vi "TLB Native Dynamic Events ver 0.17a.vi"() -> ()   [LabVIEW 2018]
uses:
  Labview Training Phase 2/Enum Controls/States for Action Engine.ctl
  TLB Type Definitions/State Type Definitions, for 0.26d versions and later.ctl
  TLB Type Definitions/Intruction Type Definitions.ctl
  TLB Type Definitions/Encoder cluster.ctl
  TLB Type Definitions/PING CLUSTER.ctl
  <vilib>/Studica/Studica Toolkit/NavX/NavX.lvlib
  <vilib>/Studica/Studica Toolkit/Background/DIO Channel.ctl
  Underlying VI's/NavX VI/navX type def.ctl
  <vilib>/myRIO/Instrument Drivers/Utilities/Utilities.lvlib
  <vilib>/Studica/Studica Toolkit/Background/I2C Channel.ctl
  TLB Type Definitions/Vision cluster.ctl
  <vilib>/NI_Real-Time Target Support.lvlib
  TLB Type Definitions/Stepper cluster.ctl
  Experimental VI's/Archived VI's/MOTOR CONTROL NO PID Type Def.ctl
  Underlying VI's/I2C Master VI/I2C MASTER Type Def.ctl
  Underlying VI's/I2C Master VI/I2C_MASTER_WRITE_NEW Type Def.ctl
  <vilib>/userdefined/High Color/IMAQdx.ctl
  Underlying VI's/I2C Master VI/Arduino_Interfacing.ctl
  TLB Type Definitions/Yaw Cluster.ctl
  TLB Type Definitions/Time cluster.ctl
  TLB Type Definitions/Y Stepper cluster.ctl
  Underlying VI's/Modified webcam FGV/Webcam AE.ctl
  Underlying VI's/Elasped Timer/Elapsed timer control.ctl
  Underlying VI's/Motor Control VI with PID/MOTOR CONTROL WITH PID AE DATA MODE TYPE DEF.ctl
  Underlying VI's/Motor Control VI with PID/MOTOR CONTROL WITH PID AE DIRECTION TYPE DEF.ctl
  TLB Type Definitions/IR Sensor Type Def.ctl
  <vilib>/myRIO/Common/Instrument Driver Framework/myRIO v1.0/AI/typedefs/AI Channels Enum.ctl
  <vilib>/myRIO/Common/Instrument Driver Framework/myRIO v1.0/AI/typedefs/AI Channels List.ctl
  <vilib>/Utility/RT CPU Load.ctl
panel:
  out "Left IR Sensor":dbl
  out "Obstacle detected":bool
  out "Speed & distance":T1
  out "Object Center Coordinates":cluster{"x":sgl, "y":sgl}
  out "Object detection cluster":T2
  out "Time up flag":bool
  out "Task selection":u8
  in  "Object recognition mode":enum16{"Ball", "Soap", "Gel", "Pipe", "None"}(ring)
  out "NavX Readings":T3
  out "Arduino Data":T4
  out "CPU loads":T5[](array[typedef]) {"ISR (%)" format="%#.2f"; "Idle (%)" format="%#.2f"; "Background (%)" format="%#.2f"; "Normal (%)" format="%#.2f"; "Above Normal (%)" format="%#.2f"; "High (%)" format="%#.2g"; "Timed Structures (%)" format="%#.2g"; "Time Critical (%)" format="%#.2g"; "Total (%)" format="%#.2g"}
  out "TASK ENABLE":bool
  out "Rising Edge":bool
  in  "Green LED":bool
  out "I2C Error":errorcluster
  out "State Logic":T6=enum."Startup"
  out "elements":T7[](array[typedef])
  in  "STOP TASK":bool
  in  "OK Button":bool
  in  "STOP":bool
  out "error out":errorcluster
  out "Action Queue Items":i32
  out "State Logic Queue Items":i32
  out "Action Queues items":string[](array[string])=["Hardware reset", "Software reset", ""]
  out "Action State":string
  # "System Health Status Update"
  # "VISION"
  # "TLB FRAMEWORK STATUS"
  # "Test Programme written by Calvin Loke    Dated: 28 Aug 2019\nTest Programme revised by Dr Alex See   Dated 30 Aug 2019\n\nRevision date: 20/03/2020\nProgramme version:   TLB Native Dynamic Events ver 0.14a"
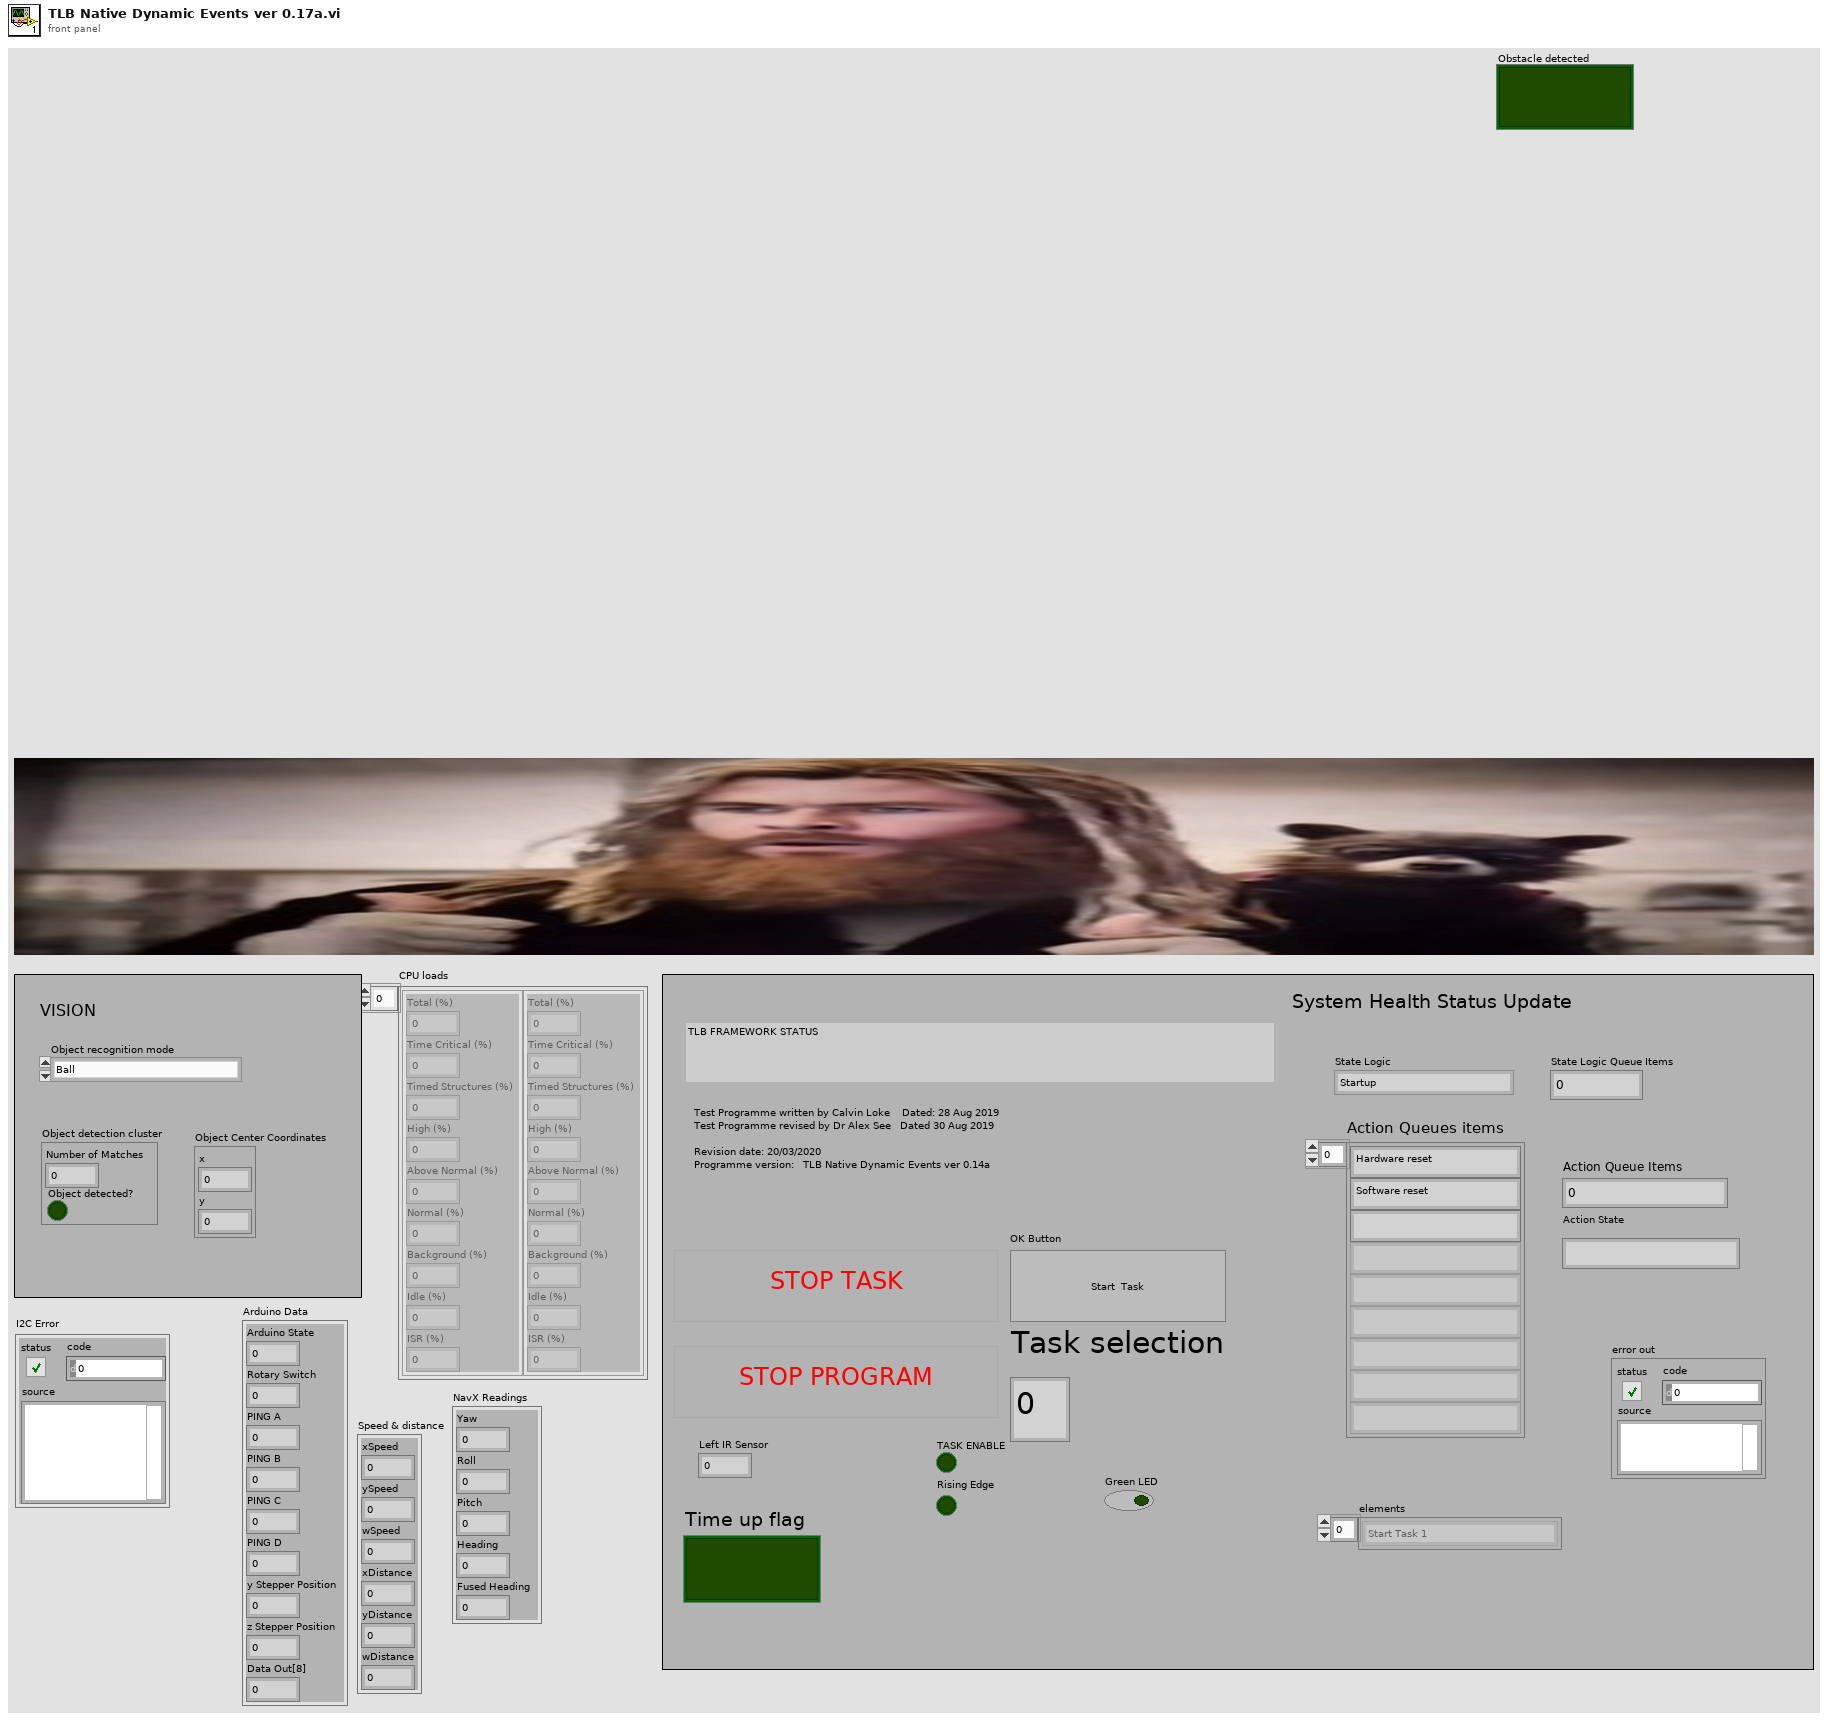
[diagram p1: front panel]
types:
  T1 = cluster{"xSpeed":dbl, "ySpeed":dbl, "wSpeed":dbl, "xDistance":dbl, "yDistance":dbl, "wDistance":dbl}
  T2 = cluster{"Number of Matches":i32, "Object detected?":bool}
  T3 = cluster{"Yaw":dbl, "Roll":dbl, "Pitch":dbl, "Heading":dbl, "Fused Heading":dbl}
  T4 = cluster{"Arduino State":u8, "Rotary Switch":u8, "PING A":u8, "PING B":u8, "PING C":u8, "PING D":u8, "y Stepper Position":u8, "z Stepper Position":u8, "Data Out[8]":u8}
  T5 = typedef "NI_Real-Time Target Support.lvlib/RT CPU Load.ctl" = cluster{"Total (%)":dbl, "Time Critical (%)":dbl, "Timed Structures (%)":dbl, "High (%)":dbl, "Above Normal (%)":dbl, "Normal (%)":dbl, "Background (%)":dbl, "Idle (%)":dbl, "ISR (%)":dbl}
  T6 = typedef "State Type Definitions.ctl" = enum16{"None", "Startup", "Move to Angle", "True Stop", "Idle", "Shutdown", "Task 1A", "Task 1B", "Task 2:Raise Arm", "Task 2:Sensor Mode", "Task 2:Reverse Mode", "Task 3", "Task 4_A", "Task 4_B", "Task 4_C", "Task 4_D", "Task 5A", "Task 5B", "Task 5C", "Task 5D", "Task 5E: POSITION ARM", "Task 5F: ARM GRAB HEIGHT", "Task 5G: CLOSE CLAW", "Task 5H: RAISE ARM", "Task 6_A", "Task 6_B", "Task 7", "Task 8A: RAISE ARM", "Task 8B: MOVE TO BOX", "Task 8C: CAM BURST", "Task 8D: PROCESS IMAGE", "Task 8E: ROBOT ADJUST", "Task 8F: CAM BURST 2", "Task 8G: PROCESS IMAGE 2", "Task 8H: ARM ADJUST", "Task 8I: ARM GRAB HEIGHT", "Task 8J: CLOSE CLAW", "Task 8K: RAISE MY SWORD", "Task 9A: Raise Arm", "Task 9B: Rotate to Angle", "Task 9C: Detect Box", "Task 9D: MOVE FORWARD", "Task 9E: MOVE LEFT", "Task 9F: SCAN IMAGE", "Task 9G: PROCESS COLOUR", "Task 9H: MOVE RIGHT", "Task 9I: SCAN IMAGE", "Task 9J: PROCESS COLOUR", "Task 9K: ROTATE 90 CW", "Task 9L: MOVE FORWARD", "Task 9M: MOVE RIGHT", "Task 9N: SCAN IMAGE", "Task 9O: PROCESS COLOUR", "Task 9P: MOVE RIGHT", "Task 9Q: SCAN IMAGE", "Task 9R: PROCESS COLOUR", "Task A1: Raise Arm", "Task A2: Rotate to Angle", "Task A3: Move Forward", "Task A4: Rotate CW 90"}
  T7 = typedef "Intruction Type Definitions.ctl" = enum16{"None", "Start Task 1", "Start Task 2", "Start Task 3", "Start Task 4", "Start Task 5", "Start Task 6", "Start Task 7", "Start Task 8 - BALL", "Start Task 8 - Gel", "Start Task 8 - Pipe", "Start Task 8 - Soap", "Start Task 9", "Start Task A", "Start Task B", "Exit"}
  T8 = typedef "IR Sensor Type Def.ctl" = cluster{"Left IR Sensor":dbl, "Arm IR Sensor":dbl, "Bottom IR Sensor":dbl}
  T9 = typedef "Y Stepper cluster.ctl" = cluster{"yStepper desired":u8}
  T10 = typedef "Time cluster.ctl" = cluster{"Time up flag":bool, "SET TIME TO CHECK":dbl}
  T11 = typedef "Yaw Cluster.ctl" = cluster{"Yaw":dbl, "Compass":dbl}
  T12 = typedef "Stepper cluster.ctl" = cluster{"y Stepper Position":u8, "z Stepper Position":u8}
  T13 = typedef "DIO Channel.ctl" = enum16{"Not Connected", "A/DIO1", "A/DIO2", "A/DIO3", "A/DIO4", "A/DIO5", "A/DIO6", "A/DIO7", "A/DIO13", "B/DIO1", "B/DIO2", "B/DIO3", "B/DIO4", "B/DIO5", "B/DIO6", "B/DIO7", "B/DIO13", "C/DIO0", "C/DIO1", "C/DIO2", "C/DIO3", "C/DIO4", "C/DIO5", "C/DIO6", "C/DIO7"}
  T14 = typedef "Vision cluster.ctl" = cluster{"Recognized Object":bool, "Object X coordinate":dbl, "Object Y coordinate":dbl}
  T15 = typedef "PING CLUSTER.ctl" = cluster{"PING_A":u8, "PING_B":u8, "PING_C":u8, "PING_D":u8}
  T16 = typedef "Encoder cluster.ctl" = cluster{"xDistance":dbl, "yDistance":dbl, "wDistance":dbl}
  T17 = cluster{"DIO Channel":T13, "FPGA VI Reference Out":refnum<k20>}
  T18 = typedef "navX type def.ctl" = enum16{"Get i2C reference", "Read Values", "Zero Yaw"}
  T19 = typedef "Arduino_Interfacing.ctl" = enum16{"Initialize", "Write to Arduino", "Read From Arduino"}
  T20 = typedef "I2C Channel.ctl" = enum16{"Not Connected", "A", "B"}
  T21 = typedef "States for Action Engine.ctl" = enum16{"Initialize", "Write", "Read"}
  T22 = cluster{"I2C Ref Out":cluster{"I2C Channel":T20, "FPGA VI Reference Out":refnum<k20>}, "Connected":bool, "Slave Address (7-bit)":u8, "Registry":u8[]}
  T23 = typedef "IMAQ Image.ctl" = refnum<image>
  T24 = typedef "State Type Definitions.ctl" = enum16{"None", "Startup", "Move to Angle", "True Stop", "Idle", "Shutdown", "Task 1", "Task 2:Raise Arm", "Task 2:Sensor Mode", "Task 2:Reverse Mode", "Task 3", "Task 4_A", "Task 4_B", "Task 4_C", "Task 4_D", "Task 5_A", "Task 5 _B", "Task 5_C", "Task 5_D", "Task 5_D_Error", "Task 5D_Error_Right", "Task 5D_Error_Left", "Task 5_E", "Task 5_F", "Task 5F_Error", "Task 5G", "Task 5H", "Task 5I", "Task 6_A", "Task 6_B", "Task 7", "Task 8", "Task 9A: Raise Arm", "Task 9B: Rotate to Angle", "Task 9C: Rotation alignmnet", "Task B"}
  T25 = typedef "MOTOR CONTROL WITH PID AE DIRECTION TYPE DEF.ctl" = enum16{"y-axis movement", "x-axis movement", "rotation", "stop", "reset encoders"}
  T26 = typedef "MOTOR CONTROL WITH PID AE DATA MODE TYPE DEF.ctl" = enum16{"Init AE", "Write to AE", "Read from AE"}
  T27 = typedef "Elapsed timer control.ctl" = enum16{"Start", "Pause", "Initialize"}
  T28 = typedef "I2C_MASTER_WRITE_NEW Type Def.ctl" = enum16{"Ultrasonic sensors", "Stepper origin", "zStepper 13.3k", "zStepper 13k", "zStepper 12k", "zStepper 11k", "zStepper 10k", "zStepper 9k", "zStepper 8k", "zStepper 7k", "zStepper 6k", "zStepper 5k", "zStepper 4k", "zStepper 3k", "zStepper 2k", "zStepper 1k", "zStepper 900", "zStepper 800", "zStepper 700", "zStepper 600", "zStepper 500", "zStepper 400", "zStepper 300", "zStepper 200", "zStepper 100", "zStepper 0", "yStepper control", "Open Claw", "Close Claw", "Soft Reset"}
  T29 = typedef "Webcam AE.ctl" = enum16{"Initialize Camera", "Open Camera", "Continuous Acquisition", "Close Camera", "Retrieve Image", "Dispose Camera Image Buffer"}
  T30 = typedef "IMAQdx.ctl" = refnum<k21>
  T31 = typedef "Webcam AE.ctl" = enum16{"Initialize Camera", "Open Camera", "Continuous Acquisition", "Close Camera", "Retrieve Image", "Dispose Image Buffers"}
  T32 = typedef "MOTOR CONTROL NO PID Type Def.ctl" = enum16{"Init", "Front Back", "Left Right", "Rotate", "Stop", "Latch"}
  T33 = typedef "AI Channels List.ctl" = T34[]
  T34 = typedef "AI Channels Enum.ctl" = enum16{"Not Connected", "AudioIn/Left", "AudioIn/Right", "C/AI0", "C/AI1", "A/AI0", "A/AI1", "A/AI2", "A/AI3", "A/AI4", "A/AI5", "A/AI6", "A/AI7", "B/AI0", "B/AI1", "B/AI2", "B/AI3", "B/AI4", "B/AI5", "B/AI6", "B/AI7", "AI/AI0", "AI/AI1", "AI/AI2", "AI/AI3", "A/AI0 (DIFF)", "A/AI1 (DIFF)", "A/AI2 (DIFF)", "A/AI3 (DIFF)", "B/AI0 (DIFF)", "B/AI1 (DIFF)", "B/AI2 (DIFF)", "B/AI3 (DIFF)"}
  T35 = typedef "I2C MASTER Type Def.ctl" = enum16{"Last State", "Mode 0", "Mode 1", "Mode 2", "Mode 3", "Mode 4", "Mode 5", "Mode 6", "Mode 7", "Mode 8", "Mode 9", "Mode 10"}
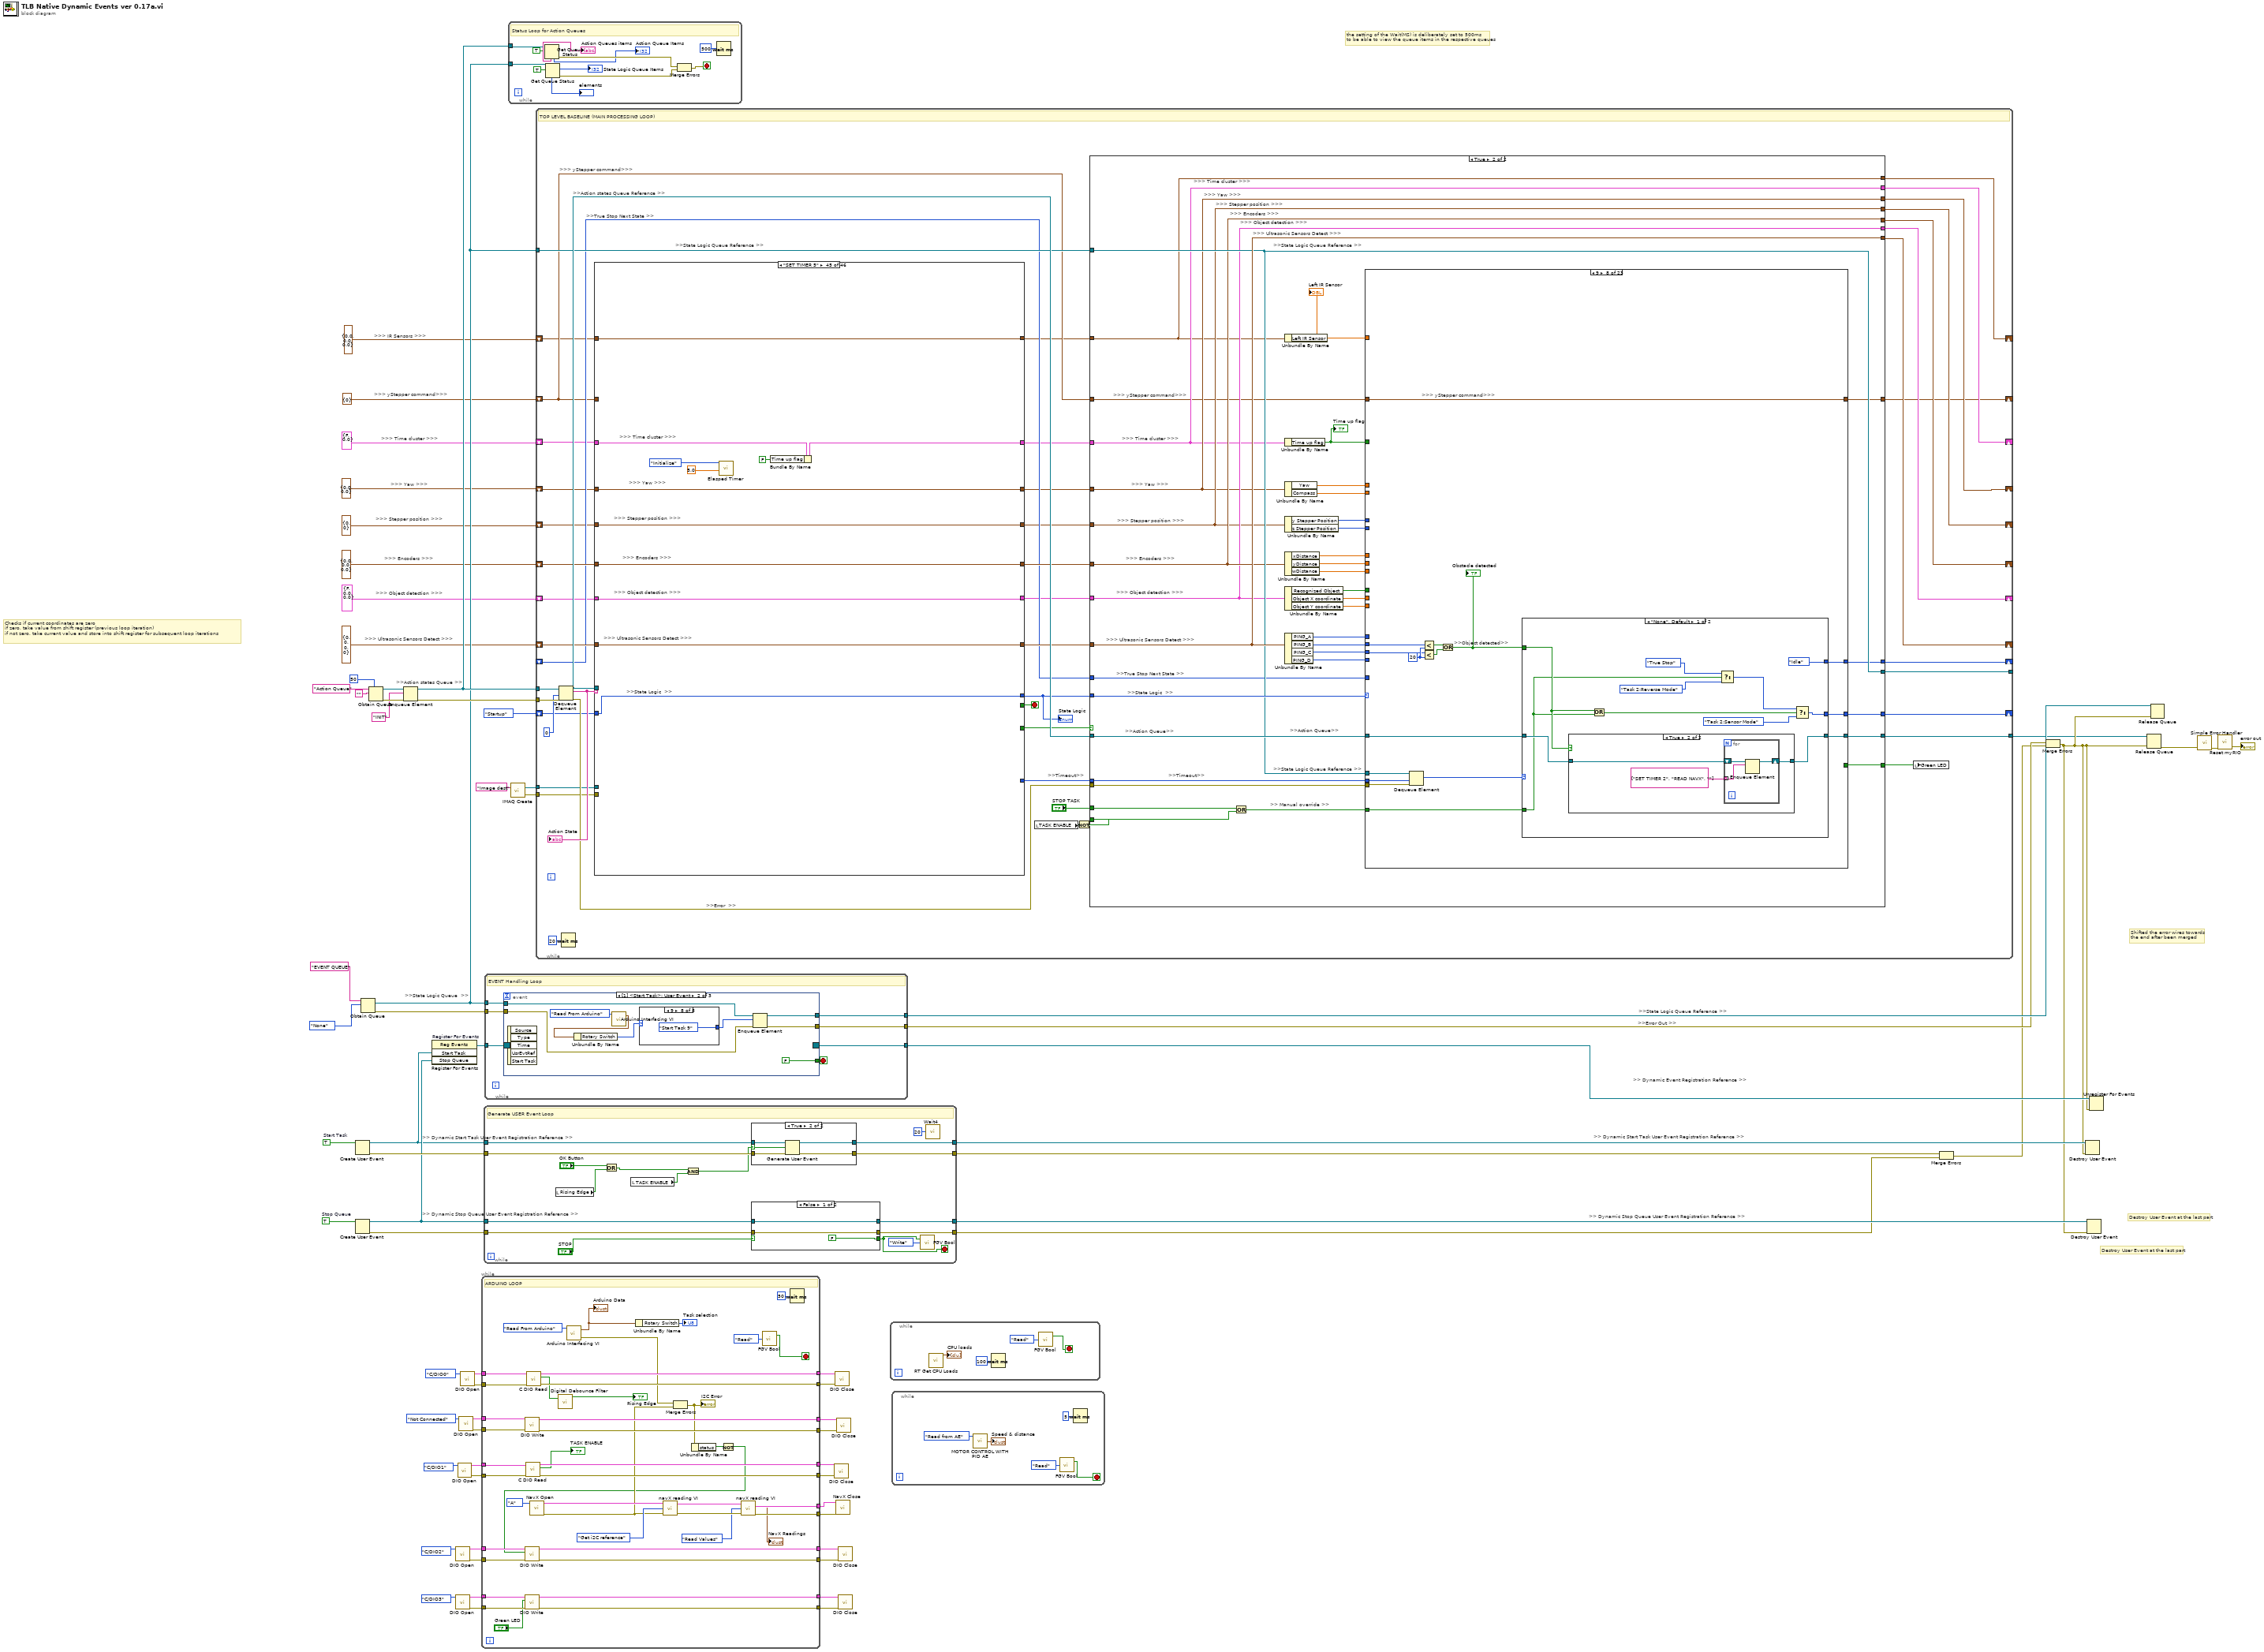
[diagram p0: block diagram]
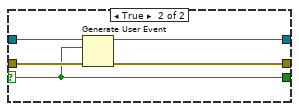
[diagram p2: hidden frame]
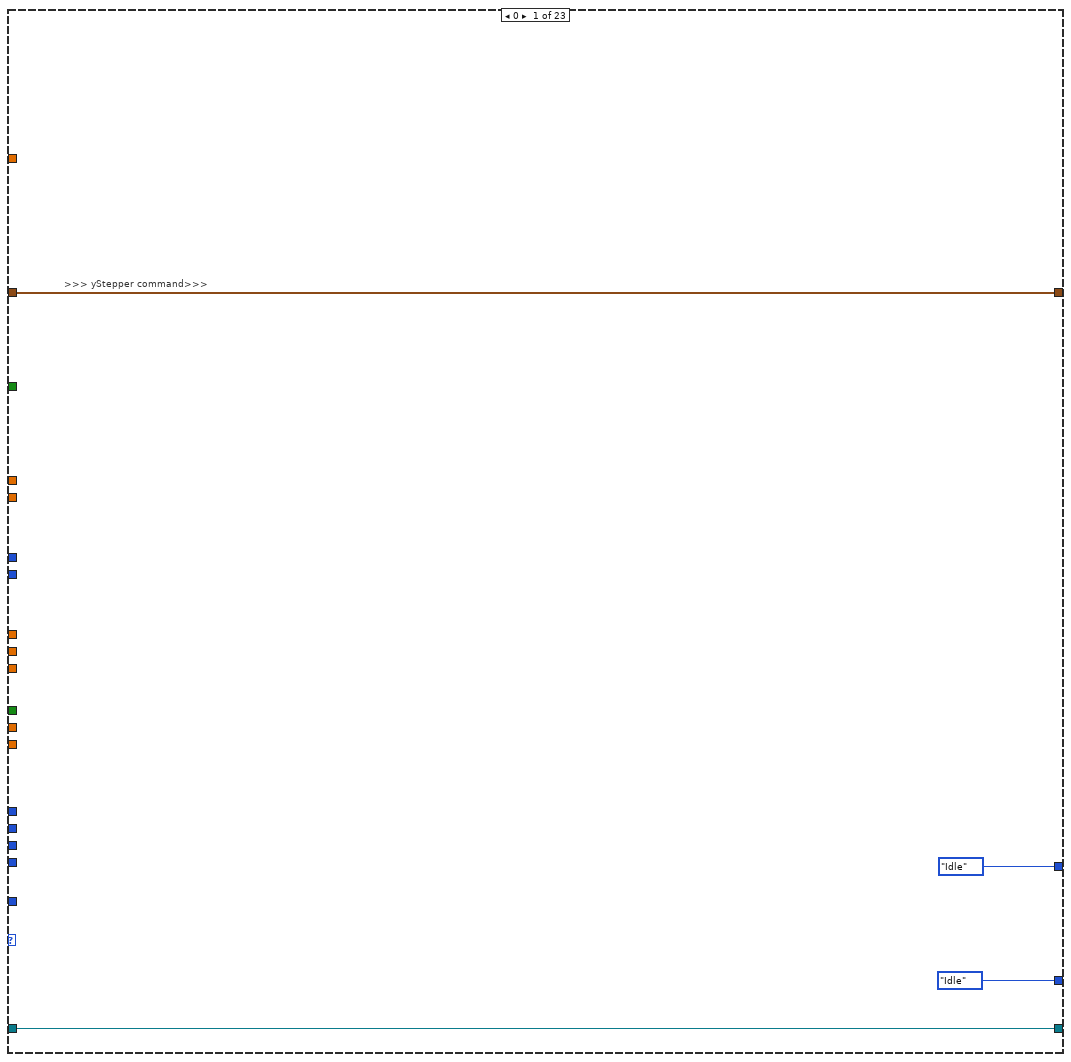
[diagram p5: hidden frame]
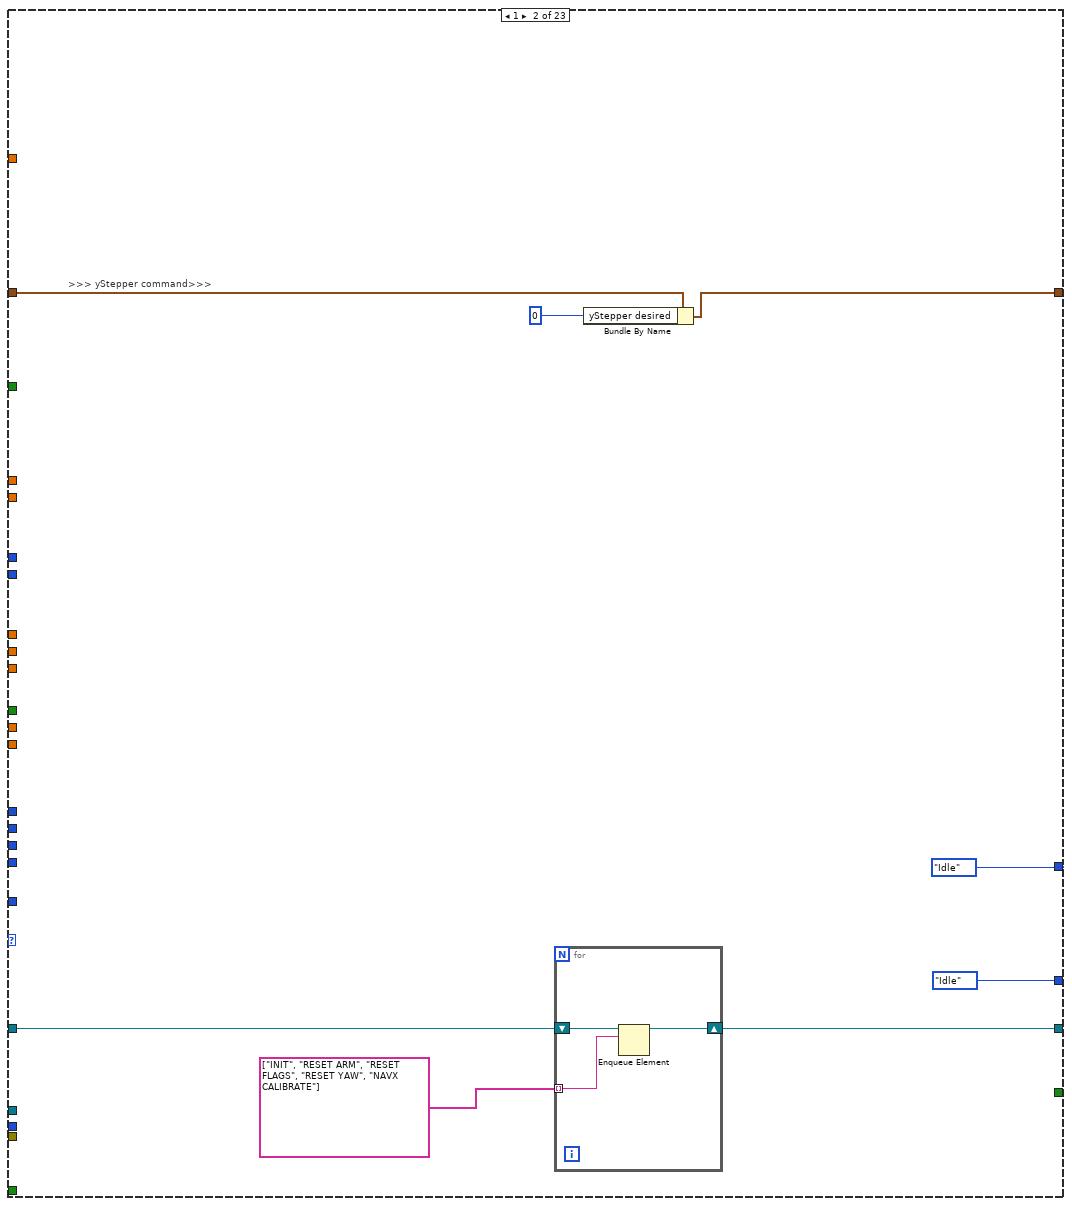
[diagram p6: hidden frame]
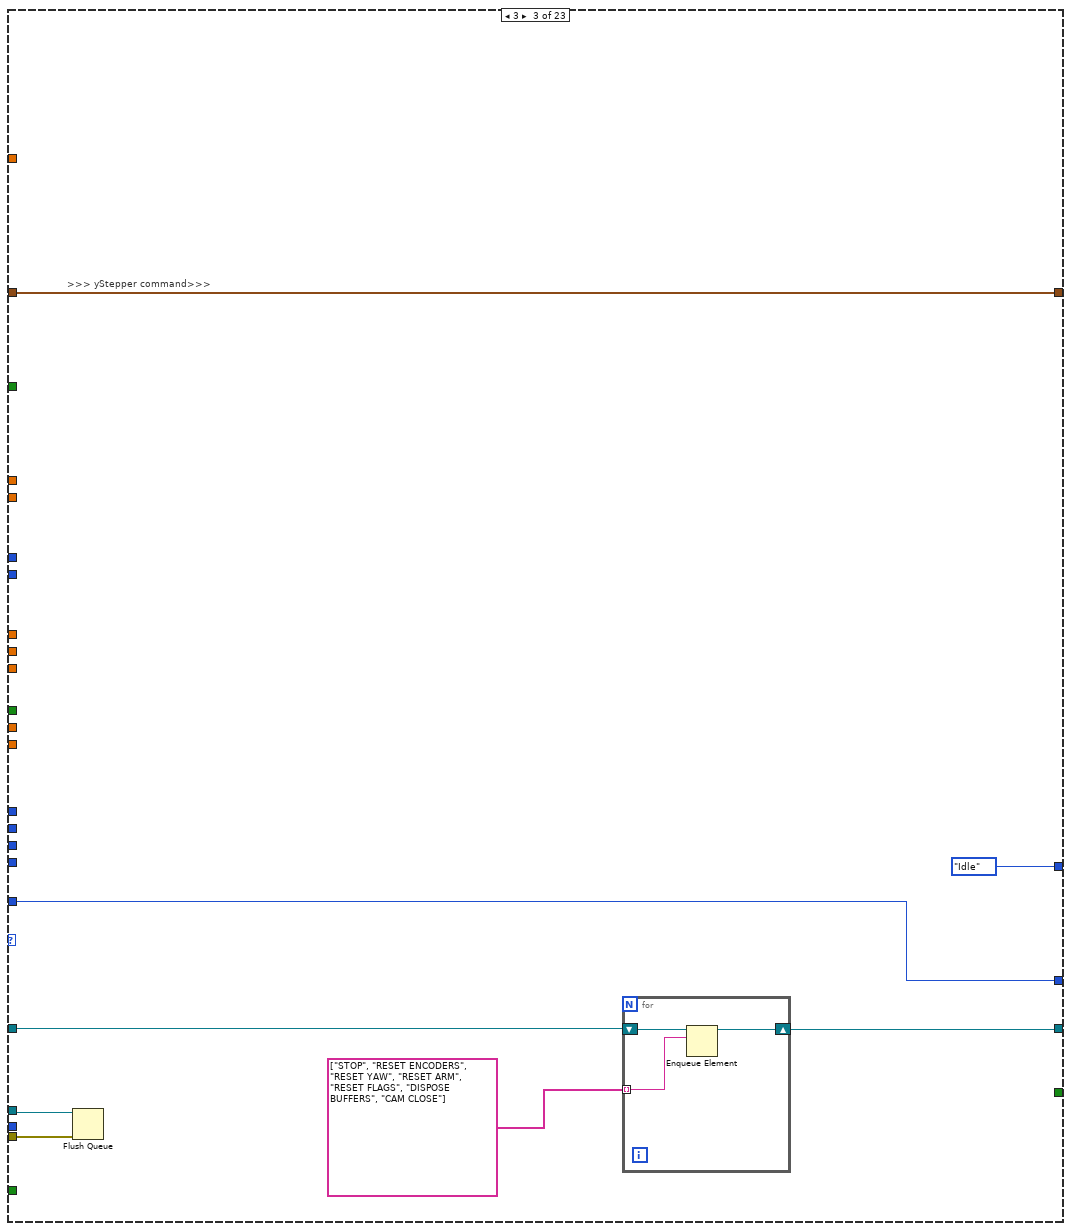
[diagram p7: hidden frame]
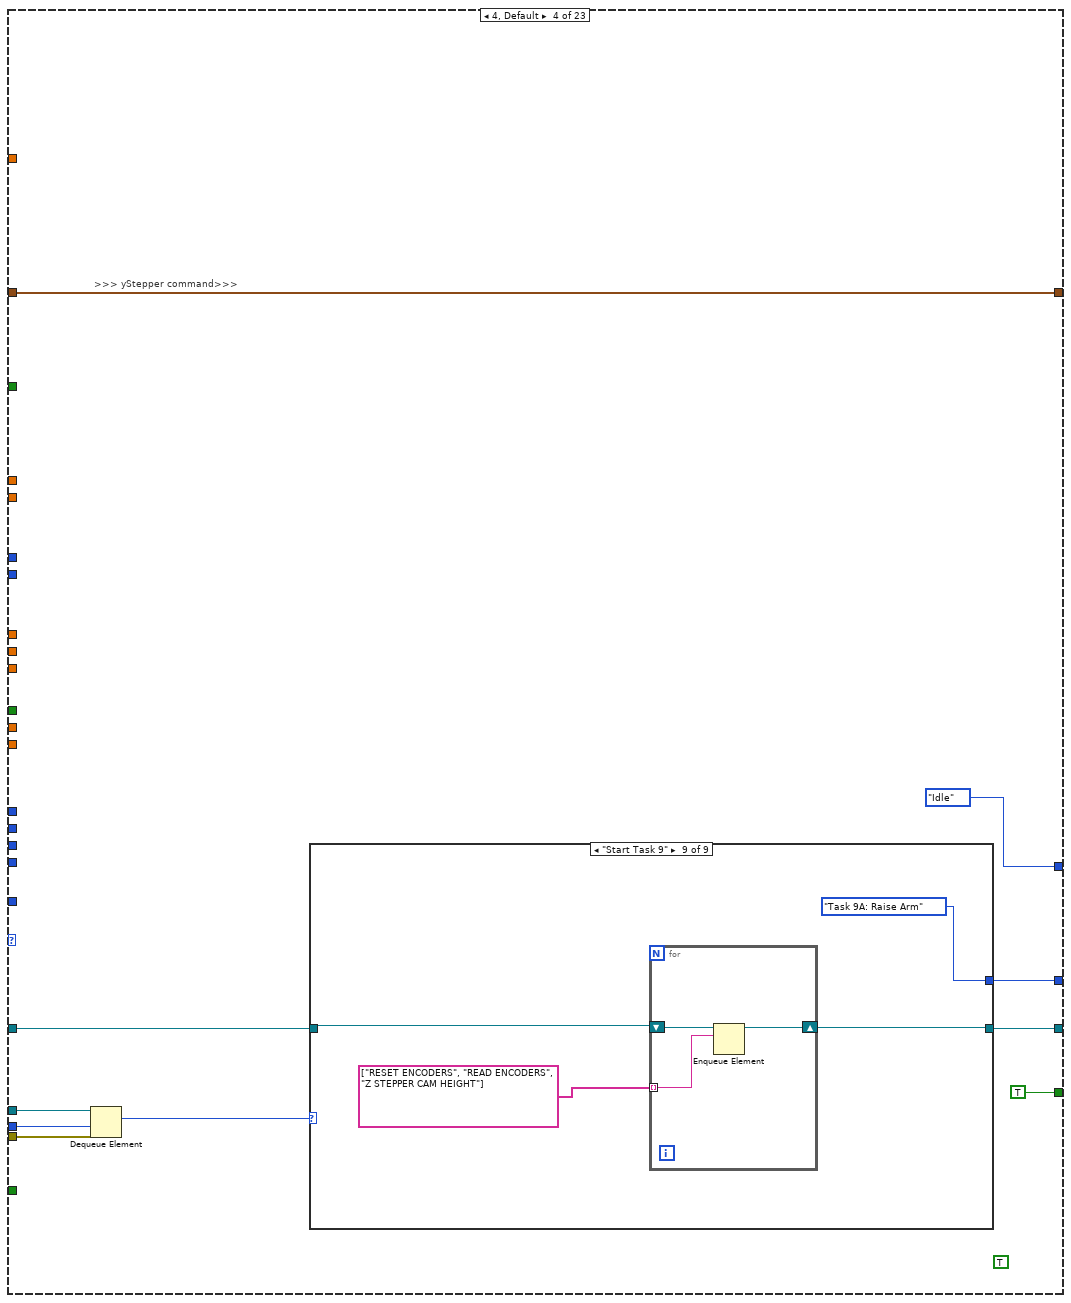
[diagram p8: hidden frame]
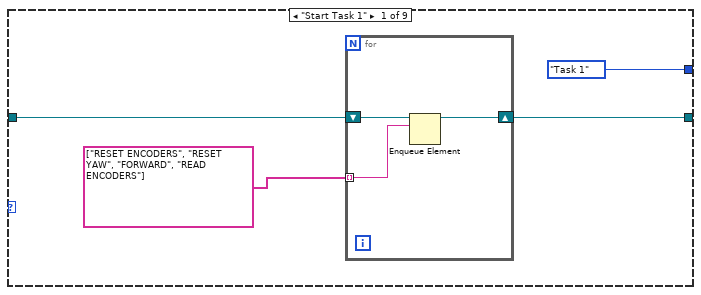
[diagram p9: hidden frame]
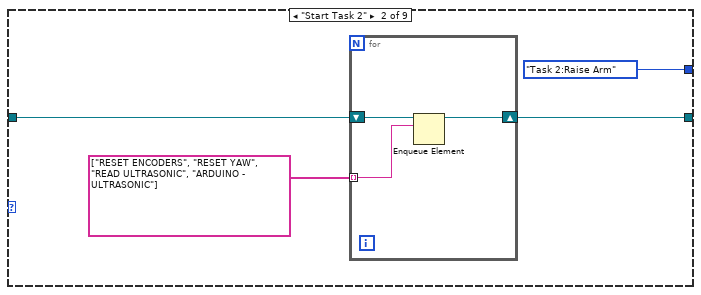
[diagram p10: hidden frame]
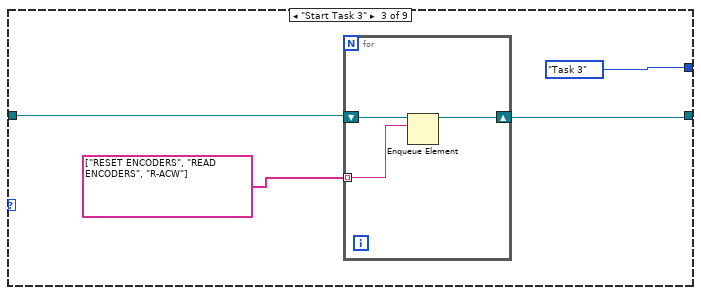
[diagram p11: hidden frame]
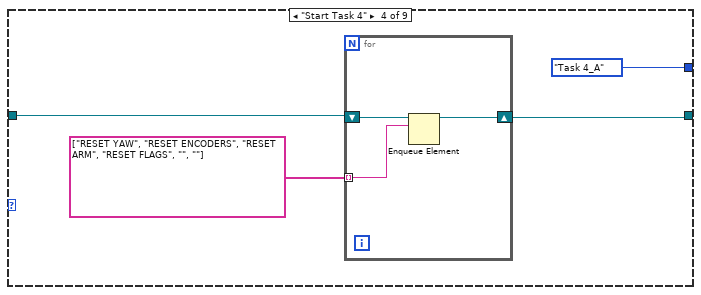
[diagram p12: hidden frame]
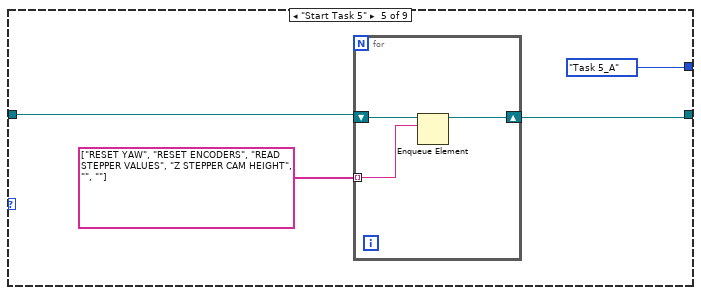
[diagram p13: hidden frame]
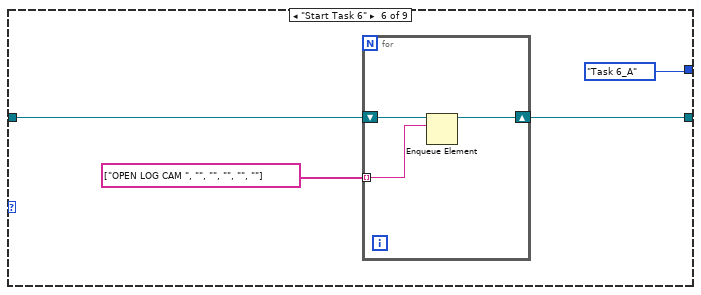
[diagram p14: hidden frame]
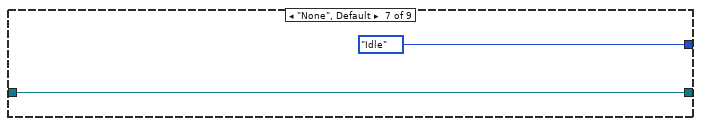
[diagram p15: hidden frame]
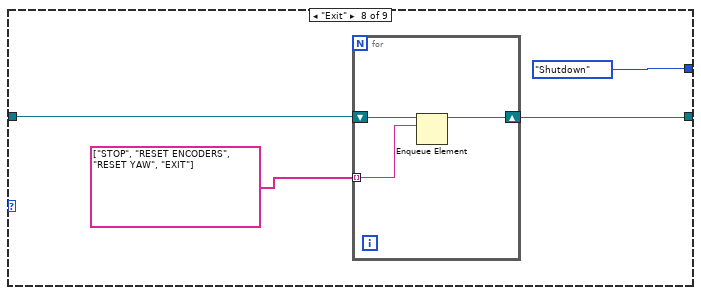
[diagram p16: hidden frame]
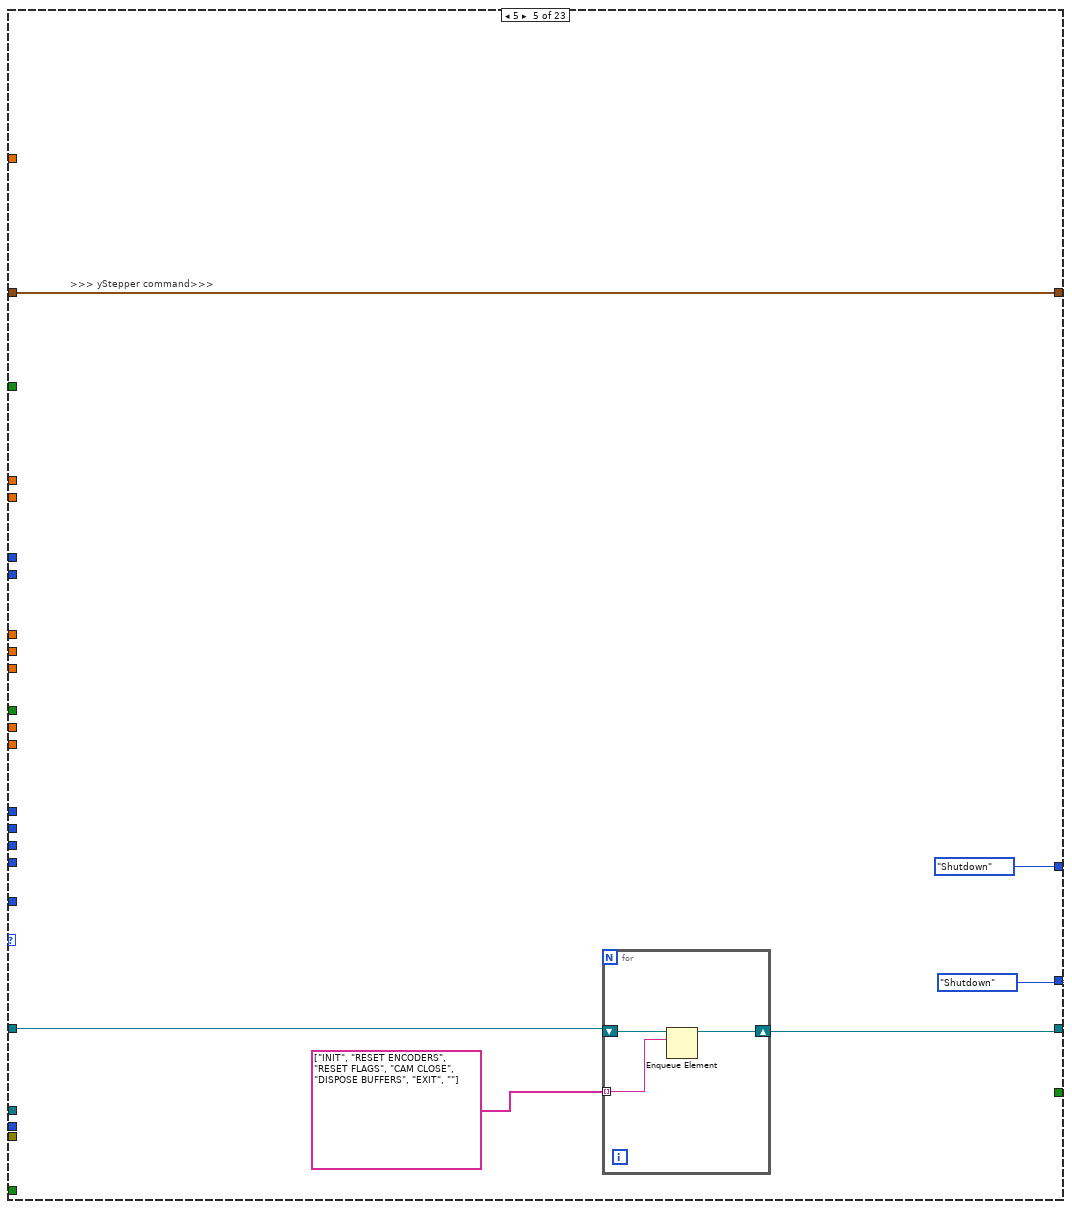
[diagram p17: hidden frame]
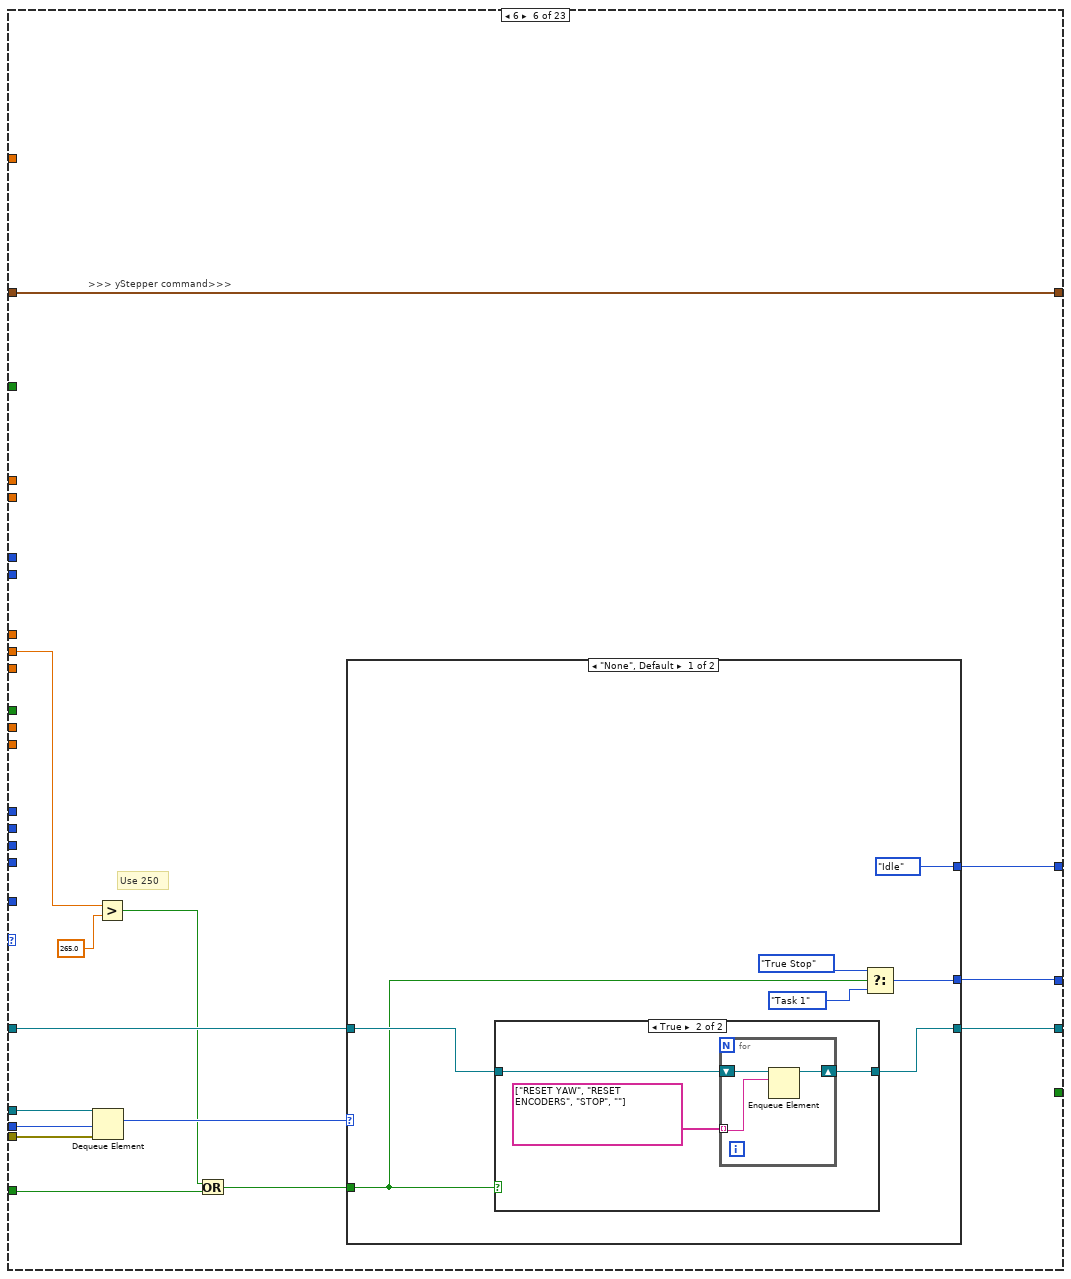
[diagram p18: hidden frame]
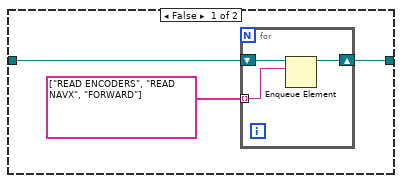
[diagram p19: hidden frame]
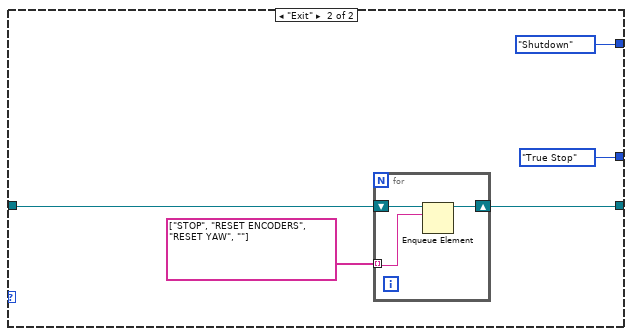
[diagram p20: hidden frame]
diagram:
  w71 = TRUE  # Stop Queue
  w70 = TRUE  # Start Task
  # ">>> IR Sensors >>>"
  # "Checks if current coordinates are zero\nif zero, take value from shift register (previous loop iteration)\nif not zero, take current value and store into shift register for subsequent loop iterations"
  # ">>> yStepper command>>>"
  # ">>> Time cluster >>>"
  # ">>> Yaw >>>"
  # ">>> Stepper position >>>"
  # ">>> Encoders >>>"
  # ">>> Object detection >>>"
  # ">>> Ultrasonic Sensors Detect >>>"
  # "the setting of the Wait(MS) is deliberately set to 500ms\nto be able to view the queue items in the respective queues"
  # ">>Error Out >>"
  # ">> Dynamic Stop Queue User Event Registration Reference >>"
  # ">> Dynamic Start Task User Event Registration Reference >>"
  # ">> Dynamic Stop Queue User Event Registration Reference >>"
  # ">> Dynamic Start Task User Event Registration Reference >>"
  # ">> Dynamic Event Registration Reference >>"
  # ">>Action states Queue >>"
  # ">>State Logic Queue  >>"
  # ">>State Logic Queue Reference >>"
  # "Destroy User Event at the last part"
  # "Destroy User Event at the last part"
  # "Shifted the error wires towards\nthe end after been merged"
  n1 = Create User Event(user event datatype=w70) -> (user event=w62:refnum<user-event>, error out=w67:errorcluster)  [unwired: 1 in]
  n2 = Create User Event(user event datatype=w71) -> (user event=w63:refnum<user-event>, error out=w66:errorcluster)  [unwired: 1 in]
  n3 = Obtain Queue(name (unnamed)="EVENT QUEUE", element data type=Intruction_Type_Definitions."None" ("Enum")) -> (queue out=w48:refnum<queue>, error out=w54:errorcluster)  [unwired: 3 in, 1 out]
  n4 = Obtain Queue(max queue size (-1, unlimited)=50, name (unnamed)="Action Queue", element data type="") -> (queue out=w57:refnum<queue>, error out=w53:errorcluster)  [unwired: 2 in, 1 out]
  n5 = Enqueue Element(queue=w57, element="INIT", error in (no error)=w53) -> (queue out=w49:refnum<queue>, error out=w52:errorcluster)  [unwired: 1 in, 1 out]
  n6 = register-events "Register For Events"(w62, w63) -> (reference out=w61:refnum<event-registration>)  [unwired: 2 in, 1 out]
  n7 = call <vilib>:"DIO Open.vi"("DIO Channel"=DIO_Channel."C/DIO2") -> ("error out"=w15:errorcluster, "DIO Info Out"=w16:T17)  [unwired: 9 in]
  n8 = call <vilib>:"DIO Open.vi"("DIO Channel"=DIO_Channel."C/DIO3") -> ("error out"=w10:errorcluster, "DIO Info Out"=w11:T17)  [unwired: 9 in]
  n9 = call <vilib>:"DIO Open.vi"("DIO Channel"=DIO_Channel."C/DIO1") -> ("error out"=w26:errorcluster, "DIO Info Out"=w27:T17)  [unwired: 9 in]
  n10 = call <vilib>:"DIO Open.vi"("DIO Channel"=DIO_Channel."Not Connected") -> ("error out"=w31:errorcluster, "DIO Info Out"=w33:T17)  [unwired: 9 in]
  n11 = call <vilib>:"DIO Open.vi"("DIO Channel"=DIO_Channel."C/DIO0") -> ("error out"=w36:errorcluster, "DIO Info Out"=w39:T17)  [unwired: 9 in]
  n12 = while {
    tunnel: w39 -> [w112]
    tunnel: [w111] -> w37
    tunnel: w36 -> [w110]
    tunnel: [w109] -> w35
    tunnel: w33 -> [w106]
    tunnel: [w105] -> w32
    tunnel: w31 -> [w104]
    tunnel: [w103] -> w30
    tunnel: [w102] -> w28
    tunnel: w27 -> [w101]
    tunnel: w26 -> [w100]
    tunnel: [w99] -> w25
    tunnel: w16 -> [w93]
    tunnel: w15 -> [w92]
    tunnel: [w91] -> w14
    tunnel: [w90] -> w13
    tunnel: w11 -> [w89]
    tunnel: w10 -> [w88]
    tunnel: [w87] -> w9
    tunnel: [w86] -> w8
    tunnel: [w80] -> w5
    tunnel: [w79] -> w6
    stop <- w114 stop-if-true
    # "ARDUINO LOOP"
    n13 = call <vilib>:"DIO Write.vi"("error in (no error)"=w88, "Input"="Green LED", "DIO Info In"=w89) -> ("error out"=w86:errorcluster, "DIO Info Out"=w87:T17)  [unwired: 7 in]
    n14 = call <vilib>:"DIO Write.vi"("error in (no error)"=w104, "DIO Info In"=w106) -> ("error out"=w103:errorcluster, "DIO Info Out"=w105:T17)  [unwired: 8 in]
    n15 = call <vilib>:"C DIO Read.vi"("error in (no error)"=w100, "DIO Info In in"=w101) -> ("error out"=w99:errorcluster, "IN"=→"TASK ENABLE":bool, "DIO Info In out"=w102:T17)  [unwired: 7 in]
    n16 = call <vilib>:"C DIO Read.vi"("error in (no error)"=w110, "DIO Info In in"=w112) -> ("error out"=w109:errorcluster, "IN"=w108:bool, "DIO Info In out"=w111:T17)  [unwired: 7 in]
    n17 = call <vilib>:"NavX Open.vi"("I2C Channel"=I2C_Channel."A") -> ("error out"=w95:errorcluster, "NavX Info"=w97:T22)  [unwired: 9 in]
    n18 = call "Digital Debounce Filter.vi"("Boolean input"=w108) -> ("Rising Edge"=→"Rising Edge":bool)  [unwired: 1 in, 2 out]
    n19 = call "Arduino Interfacing VI.vi"("AE Mode"=Arduino_Interfacing."Read From Arduino") -> ("error out"=w83:errorcluster, "Arduino Data"=w76:T4)  [unwired: 3 in]
    "Arduino Data" <- w76
    n20 = Unbundle By Name(w76) -> ("Rotary Switch"=→"Task selection":u8)
    n21 = call "navX reading VI.vi"("NavX Info In"=w97, "Mode"=navX_type_def."Get i2C reference", "error in (no error)"=w95) -> ("NavX Info Out"=w82:T22, "Error Out"=w81:errorcluster)  [unwired: 2 out]
    n22 = Merge Errors(w83, w95) -> (w74:errorcluster)
    "I2C Error" <- w74
    n23 = Unbundle By Name(w74) -> ("status"=w73:bool)
    n24 = Not(x=w73) -> (.not. x?=w72:bool)
    n25 = call <vilib>:"DIO Write.vi"("error in (no error)"=w92, "Input"=w72, "DIO Info In"=w93) -> ("error out"=w90:errorcluster, "DIO Info Out"=w91:T17)  [unwired: 7 in]
    n26 = call "navX reading VI.vi"("NavX Info In"=w82, "Mode"=navX_type_def."Read Values", "error in (no error)"=w81) -> ("NavX Info Out"=w80:T22, "NavX Readings"=→"NavX Readings":T3, "Error Out"=w79:errorcluster)  [unwired: 1 out]
    n27 = call "FGV Bool.vi"("Init/Read/Write State"=States_for_Action_Engine."Read") -> ("Output node"=w114:bool)  [unwired: 2 in, 1 out]
    n28 = Wait (ms)(milliseconds to wait=u32 50) -> ()  [unwired: 1 out]
  }
  n29 = while {
    tunnel: w62 -> [w132]
    tunnel: w63 -> [w131]
    tunnel: [w130] -> w69
    tunnel: [w129] -> w68
    tunnel: w67 -> [w128]
    tunnel: [w127] -> w65
    tunnel: w66 -> [w126]
    tunnel: [w125] -> w64
    stop <- w123 stop-if-true
    # "Generate USER Event Loop"
    n30 = local read "Rising Edge"() -> (w119:bool)
    n31 = Or(x="OK Button", y=w119) -> (x .or. y?=w118:bool)
    n32 = local read "TASK ENABLE"() -> (w117:bool)
    n33 = And(x=w118, y=w117) -> (x .and. y?=w116:bool)
    n34 = case shown="True" w116 {
      selector: w116 -> [_ w143]
      tunnel: w132 -> [w142 w147]
      tunnel: [w142 w146] -> w129
      tunnel: w128 -> [w141 w145]
      tunnel: [w141 w144] -> w127
      frame False {
      }
      frame True {
        n35 = Generate User Event(user event=w147, event data cluster=w143, error in=w145) -> (user event out=w146:refnum<user-event>, error out=w144:errorcluster)  [unwired: 1 in]
      }
    }
    n36 = case shown="False" "STOP" {
      selector: "STOP" -> [_ w136]
      tunnel: w131 -> [w135 w140]
      tunnel: [w135 w139] -> w130
      tunnel: w126 -> [w134 w138]
      tunnel: [w134 w137] -> w125
      tunnel: [FALSE w136] -> w123
      frame False {
      }
      frame True {
        n37 = Generate User Event(user event=w140, event data cluster=w136, error in=w138) -> (user event out=w139:refnum<user-event>, error out=w137:errorcluster)  [unwired: 1 in]
      }
    }
    n38 = call "FGV Bool.vi"("Init/Read/Write State"=States_for_Action_Engine."Write", "Input Node"=w123) -> ()  [unwired: 1 in, 2 out]
    n39 = call "Wait4"("Count(uSec)"=u32 20) -> ()  [unwired: 1 out]
  }
  n40 = while {
    tunnel: w61 -> [w154]
    tunnel: [w153] -> w60
    tunnel: w48 -> [w151]
    tunnel: [w150] -> w59
    tunnel: w54 -> [w149]
    tunnel: [w148] -> w51
    stop <- w152 stop-if-true
    # "EVENT Handling Loop"
    n41 = event shown="[1] <Start Task>: User Event" {
      selector: w154 -> [_ _ _]
      dyn-events: [_ _ _] -> w153
      timeout: _ -> [_ _ _]
      tunnel: [FALSE FALSE w183] -> w152
      tunnel: w151 -> [w159 w168 w181]
      tunnel: [w158 w167 w182] -> w150
      tunnel: w149 -> [w157 w166 w180]
      tunnel: [w156 w165 w179] -> w148
      event Timeout {
        n42 = event-data() -> ()  [unwired: 1 in, 3 out]
        n43 = Enqueue Element(queue=w159, element=Intruction_Type_Definitions."None" ("Enum"), error in (no error)=w157) -> (queue out=w158:refnum<queue>, error out=w156:errorcluster)  [unwired: 1 in, 1 out]
      }
      event User Event {
        n44 = event-data() -> ()  [unwired: 1 in, 5 out]
        n45 = call "Arduino Interfacing VI.vi"("AE Mode"=Arduino_Interfacing."Read From Arduino") -> ("Arduino Data"=w162:T4)  [unwired: 3 in, 1 out]
        n46 = Unbundle By Name(w162) -> ("Rotary Switch"=w161:u8)
        n47 = case shown="9" w161 {
          tunnel: [Intruction_Type_Definitions."None" ("Enum") Intruction_Type_Definitions."Start Task 1" ("Enum") Intruction_Type_Definitions."Start Task 2" ("Enum") Intruction_Type_Definitions."Start Task 3" ("Enum") Intruction_Type_Definitions."Start Task 4" ("Enum") Intruction_Type_Definitions."Start Task 5" ("Enum") Intruction_Type_Definitions."Start Task 6" ("Enum") Intruction_Type_Definitions."Start Task 9" ("Enum")] -> w164
          frame 0, Default {
          }
          frame 1 {
          }
          frame 2 {
          }
          frame 3 {
          }
          frame 4 {
          }
          frame 5 {
          }
          frame 6 {
          }
          frame 9 {
          }
        }
        n48 = Enqueue Element(queue=w168, element=w164, error in (no error)=w166) -> (queue out=w167:refnum<queue>, error out=w165:errorcluster)  [unwired: 1 in, 1 out]
      }
      event User Event {
        n49 = event-data() -> ("Stop Queue"=w183:bool)  [unwired: 1 in, 4 out]
        n50 = Enqueue Element At Opposite End(queue=w181, element=Intruction_Type_Definitions."Exit" ("Enum"), error in (no error)=w180) -> (queue out=w182:refnum<queue>, error out=w179:errorcluster)  [unwired: 1 in, 1 out]
      }
    }
  }
  n51 = while {
    tunnel: w49 -> [w193]
    tunnel: w48 -> [w190]
    stop <- w187 stop-if-true
    # "Status Loop for Action Queues"
    n52 = Get Queue Status(queue=w193, return elements? (F)=TRUE) -> (error out=w189:errorcluster, # elements in queue=→"Action Queue Items":i32, elements=→"Action Queues items":string[])  [unwired: 1 in, 5 out]
    n53 = Get Queue Status(queue=w190, return elements? (F)=TRUE) -> (# pending remove=→"State Logic Queue Items":i32, error out=w188:errorcluster, elements=→"elements":T7[])  [unwired: 1 in, 5 out]
    n54 = Merge Errors(w189, w188) -> (w187:errorcluster)
    n55 = Wait (ms)(milliseconds to wait=u32 500) -> ()  [unwired: 1 out]
  }
  n56 = call "IMAQ Create"("Image Name"="Image dest") -> ("New Image"=w20:T23, "error out"=w19:errorcluster)  [unwired: 4 in]
  n57 = while {
    tunnel: w48 -> [w230]
    tunnel: w49 -> [w242]
    tunnel: w52 -> [w240]
    tunnel: [w239] -> _
    tunnel: [w238] -> w42
    shift-right: [w231] -> _
    shift-left: T15 {"PING_A"=0, "PING_B"=0, "PING_C"=0, "PING_D"=0} -> [w233]
    shift-right: [w224] -> _
    shift-left: State_Type_Definitions."Startup" ("Enum") -> [w227]
    shift-right: [w220] -> _
    shift-left: T16 {"xDistance"=0.0, "yDistance"=0.0, "wDistance"=0.0} -> [w222]
    shift-right: [w217] -> _
    shift-left: _ -> [w216]
    tunnel: w20 -> [w215]
    tunnel: w19 -> [w214]
    shift-right: [w211] -> _
    shift-left: T14 {"Recognized Object"=FALSE, "Object X coordinate"=0.0, "Object Y coordinate"=0.0} -> [w213]
    shift-right: [w208] -> _
    shift-left: T12 {"y Stepper Position"=0, "z Stepper Position"=0} -> [w210]
    shift-right: [w205] -> _
    shift-left: T11 {"Yaw"=0.0, "Compass"=0.0} -> [w207]
    shift-right: [w202] -> _
    shift-left: T10 {"Time up flag"=FALSE, "SET TIME TO CHECK"=0.0} -> [w204]
    shift-right: [w200] -> _
    shift-left: T9 {"yStepper desired"=0} -> [w201]
    shift-right: [w196] -> _
    shift-left: T8 {"Left IR Sensor"=0.0, "Arm IR Sensor"=0.0, "Bottom IR Sensor"=0.0} -> [w198]
    stop <- w229 stop-if-true
    # ">>> yStepper command>>>"
    # ">>True Stop Next State >>"
    # ">>Error  >>"
    # ">>Timeout>>"
    # ">>Action states Queue Reference >>"
    # ">>State Logic Queue Reference >>"
    # "TOP LEVEL BASELINE (MAIN PROCESSING LOOP)"
    n58 = Dequeue Element(queue=w242, timeout in ms (-1)=0, error in (no error)=w240) -> (queue out=w234:refnum<queue>, element=w241:string, error out=w235:errorcluster)  [unwired: 1 out]
    "Action State" <- w241
    n59 = Wait (ms)(milliseconds to wait=u32 20) -> ()  [unwired: 1 out]
    n60 = case shown="\"SET TIMER 5\"" w241 {
      tunnel: [_ _ _ _ _ _ _ _ _ _ _ _ _ _ _ _ _ _ 0 w1421 _ _ _ _ _ _ _ _ _ _ _ _ _ _ _ _ _ _ _ _ _ _ _ _ _ _] -> w237
      tunnel: w234 -> [_ _ _ _ _ _ _ _ _ _ _ _ _ _ _ _ _ _ _ _ _ _ _ _ _ _ _ _ _ _ _ _ _ _ _ _ _ _ _ _ _ _ _ _ _ _]
      tunnel: w233 -> [w1192 w1201 w1213 w1224 w1241 w1252 w1263 w1275 w1287 w1298 w1305 w1320 w1334 w1346 w1354 w1366 w1391 w1401 w1412 w1422 w1431 w1441 w1471 w1482 w1490 w1499 w1512 w1525 w1535 w1544 w1561 w1570 w1581 w1591 w1601 w1611 w1618 w1630 w1646 w1652 w1664 w1676 w1688 w1700 w1712 w1723]
      tunnel: [w1192 w1201 w1213 w1224 w1241 w1252 w1263 w1275 w1287 w1298 w1305 w1320 w1335 w1346 w1354 w1366 w1392 w1401 w1412 w1422 w1431 w1441 w1470 w1482 w1490 w1499 w1512 w1525 w1535 w1544 w1561 w1570 w1581 w1591 w1601 w1611 w1618 w1630 w1646 w1652 w1664 w1676 w1688 w1700 w1712 w1723] -> w232
      tunnel: [TRUE TRUE _ _ _ _ _ _ _ _ _ _ _ _ _ _ _ _ _ _ _ _ _ _ _ _ _ _ _ _ _ _ _ _ _ _ _ _ _ _ _ _ _ _ _ _] -> w229
      tunnel: w227 -> [w1190 w1199 w1212 w1223 w1240 w1251 w1262 w1274 w1286 w1297 w1304 w1319 w1333 w1345 w1352 w1365 w1390 w1400 w1409 w1419 w1430 w1440 w1469 w1481 w1489 w1498 w1511 w1524 w1534 w1543 w1560 w1569 w1580 w1590 w1600 w1610 w1617 w1629 w1645 w1651 w1663 w1675 w1687 w1699 w1711 w1722]
      tunnel: [_ _ _ _ _ _ _ _ _ _ _ _ _ _ _ _ _ _ _ TRUE _ _ _ _ _ _ _ _ _ _ _ _ _ _ _ _ _ _ _ _ _ _ _ _ _ _] -> w226
      tunnel: [w1190 w1199 w1212 w1223 w1240 w1251 w1262 w1274 w1286 w1297 w1304 w1319 w1333 w1345 w1352 w1365 w1390 w1400 w1409 w1419 w1430 w1440 w1469 w1481 w1489 w1498 w1511 w1524 w1534 w1543 w1560 w1569 w1580 w1590 w1600 w1610 w1617 w1629 w1645 w1651 w1663 w1675 w1687 w1699 w1711 w1722] -> w225
      tunnel: w222 -> [w1189 w1198 w1211 w1226 w1239 w1250 w1261 w1273 w1285 w1296 w1306 w1318 w1332 w1347 w1356 w1367 w1389 w1402 w1408 w1418 w1432 w1442 w1459 w1480 w1492 w1500 w1513 w1526 w1536 w1545 w1562 w1572 w1583 w1593 w1603 w1613 w1620 w1632 w1648 w1654 w1666 w1678 w1690 w1702 w1714 w1725]
      tunnel: [w1189 w1198 w1211 w1226 w1239 w1250 w1261 w1273 w1285 w1296 w1306 w1317 w1332 w1347 w1356 w1367 w1388 w1402 w1408 w1418 w1432 w1442 w1458 w1480 w1492 w1500 w1513 w1526 w1536 w1545 w1562 w1572 w1583 w1593 w1603 w1613 w1620 w1632 w1648 w1654 w1666 w1678 w1690 w1702 w1714 w1725] -> w221
      tunnel: w215 -> [w1184 _ _ _ _ _ _ _ _ _ _ _ _ _ _ _ _ _ _ _ _ _ _ _ _ _ _ _ _ _ w1556 _ _ _ _ _ _ _ _ _ _ _ _ _ _ _]
      tunnel: w214 -> [_ _ _ _ _ _ _ _ _ _ _ _ _ _ _ _ _ _ _ _ _ _ _ _ _ _ _ _ w1528 _ w1558 w1568 _ _ _ _ _ _ _ _ _ _ _ _ _ _]
      tunnel: w213 -> [w1188 w1197 w1210 w1225 w1238 w1249 w1260 w1272 w1284 w1294 w1303 w1316 w1331 w1340 w1355 w1364 w1380 w1399 w1407 w1417 w1429 w1439 w1464 w1478 w1491 w1497 w1510 w1523 w1530 w1542 w1553 w1571 w1582 w1592 w1602 w1612 w1619 w1631 w1647 w1653 w1665 w1677 w1689 w1701 w1713 w1724]
      tunnel: [w1188 w1197 w1210 w1225 w1238 w1249 w1260 w1272 w1284 w1294 w1303 w1316 w1331 w1340 w1355 w1364 w1379 w1399 w1407 w1417 w1429 w1439 w1463 w1478 w1491 w1497 w1510 w1523 w1530 w1542 w1552 w1571 w1582 w1592 w1602 w1612 w1619 w1631 w1647 w1653 w1665 w1677 w1689 w1701 w1713 w1724] -> w212
      tunnel: w210 -> [w1187 w1196 w1209 w1227 w1237 w1248 w1259 w1271 w1283 w1293 w1302 w1315 w1330 w1348 w1357 w1363 w1385 w1398 w1406 w1416 w1428 w1438 w1454 w1477 w1488 w1496 w1509 w1522 w1533 w1541 w1563 w1573 w1579 w1589 w1599 w1609 w1621 w1633 w1644 w1655 w1667 w1679 w1691 w1703 w1715 w1726]
      tunnel: [w1187 w1196 w1209 w1227 w1237 w1248 w1259 w1271 w1283 w1293 w1302 w1315 w1330 w1348 w1357 w1363 w1384 w1398 w1406 w1416 w1428 w1438 w1453 w1477 w1488 w1496 w1509 w1522 w1533 w1541 w1563 w1573 w1579 w1589 w1599 w1609 w1621 w1633 w1643 w1655 w1667 w1679 w1691 w1703 w1715 w1726] -> w209
      tunnel: w207 -> [w1186 w1195 w1207 w1228 w1235 w1246 w1258 w1269 w1281 w1292 w1301 w1314 w1323 w1343 w1358 w1362 w1375 w1397 w1405 w1415 w1427 w1437 w1450 w1476 w1485 w1495 w1508 w1521 w1532 w1540 w1564 w1574 w1578 w1586 w1596 w1606 w1622 w1634 w1638 w1656 w1668 w1680 w1692 w1704 w1716 w1727]
      tunnel: [w1186 w1195 w1207 w1228 w1235 w1246 w1258 w1269 w1281 w1292 w1301 w1314 w1323 w1342 w1358 w1362 w1374 w1397 w1405 w1415 w1427 w1437 w1449 w1476 w1485 w1495 w1508 w1521 w1532 w1540 w1564 w1574 w1578 w1586 w1596 w1606 w1622 w1634 w1638 w1656 w1668 w1680 w1692 w1704 w1716 w1727] -> w206
      tunnel: w204 -> [w1183 w1194 w1208 w1229 w1236 w1247 w1257 w1270 w1282 w1291 w1300 w1313 w1322 w1339 w1359 w1361 w1371 w1394 w1404 w1414 w1426 w1436 w1447 w1474 w1484 w1494 w1507 w1520 w1531 w1539 w1565 w1575 w1577 w1585 w1595 w1605 w1623 w1635 w1637 w1650 w1662 w1674 w1686 w1698 w1710 w1721]
      tunnel: [w1183 w1194 w1208 w1229 w1236 w1247 w1257 w1270 w1282 w1291 w1300 w1313 w1322 w1339 w1359 w1361 w1371 w1394 w1404 w1414 w1426 w1436 w1446 w1474 w1484 w1494 w1507 w1520 w1531 w1539 w1565 w1575 w1577 w1585 w1595 w1605 w1623 w1635 w1637 w1650 w1660 w1672 w1684 w1696 w1708 w1720] -> w203
      tunnel: w201 -> [_ _ _ _ _ _ _ _ _ _ _ _ _ _ _ _ _ _ _ _ _ _ _ _ _ _ _ _ _ _ _ _ _ _ _ _ _ w1626 _ _ _ _ _ _ _ _]
      tunnel: [w1182 w1193 w1202 w1219 w1230 w1242 w1253 w1264 w1276 w1288 w1299 w1307 w1321 w1336 w1350 w1360 w1368 w1393 w1403 w1413 w1425 w1433 w1443 w1473 w1483 w1493 w1501 w1514 w1527 w1537 w1546 w1566 w1576 w1584 w1594 w1604 w1614 w1624 w1636 w1649 w1657 w1669 w1681 w1693 w1705 w1717] -> w197
      tunnel: w198 -> [w1182 w1193 w1202 w1219 w1230 w1242 w1253 w1264 w1276 w1288 w1299 w1307 w1321 w1336 w1351 w1360 w1368 w1393 w1403 w1413 w1425 w1433 w1443 w1473 w1483 w1493 w1501 w1514 w1527 w1537 w1546 w1566 w1576 w1584 w1594 w1604 w1614 w1624 w1636 w1649 w1657 w1669 w1681 w1693 w1705 w1717]
      frame "Exit" {
        # ">>State Logic  >>"
        # ">>> Time cluster >>>"
        # ">>> Yaw >>>"
        # ">>> Stepper position >>>"
        # ">>> Encoders >>>"
        # ">>> Object detection >>>"
        # ">>> Ultrasonic Sensors Detect >>>"
        n61 = call "Imaq Dispose"("All Images? (No)"=TRUE, "Image"=w1184) -> ()  [unwired: 4 in, 1 out]
      }
      frame "----Movement States----" {
        # ">>State Logic  >>"
        # ">>> Time cluster >>>"
        # ">>> Yaw >>>"
        # ">>> Stepper position >>>"
        # ">>> Encoders >>>"
        # ">>> Object detection >>>"
        # ">>> Ultrasonic Sensors Detect >>>"
      }
      frame "FORWARD" {
        # ">>State Logic  >>"
        # ">>> Time cluster >>>"
        # ">>> Yaw >>>"
        # ">>> Stepper position >>>"
        # ">>> Encoders >>>"
        # ">>> Object detection >>>"
        # ">>> Ultrasonic Sensors Detect >>>"
        n62 = Unbundle By Name(w1207) -> ("Yaw"=w1203:dbl)
        n63 = call "MOTOR CONTROL WITH PID AE.vi"("Yaw"=w1203, "Speed"=50.0, "Direction"=MOTOR_CONTROL_WITH_PID_AE_DIRECTION_TYPE_DEF."y-axis movement", "AE Mode"=MOTOR_CONTROL_WITH_PID_AE_DATA_MODE_TYPE_DEF."Write to AE") -> ()  [unwired: 1 out]
      }
      frame "FORWARD - IR ASSIST" {
        # ">>State Logic  >>"
        # ">>> Time cluster >>>"
        # ">>> Yaw >>>"
        # ">>> Stepper position >>>"
        # ">>> Encoders >>>"
        # ">>> Object detection >>>"
        # ">>> Ultrasonic Sensors Detect >>>"
        n64 = Unbundle By Name(w1219) -> ("Left IR Sensor"=w1218:dbl)
        n65 = Subtract(x=w1218, y=20.0) -> (x-y=w1216:dbl)
        n66 = Multiply(x=w1216, y=0.2) -> (x*y=w1214:dbl)
        n67 = call "MOTOR CONTROL WITH PID AE.vi"("Yaw"=w1214, "Speed"=30.0, "Direction"=MOTOR_CONTROL_WITH_PID_AE_DIRECTION_TYPE_DEF."y-axis movement", "AE Mode"=MOTOR_CONTROL_WITH_PID_AE_DATA_MODE_TYPE_DEF."Write to AE") -> ()  [unwired: 1 out]
      }
      frame "LEFT" {
        # ">>State Logic  >>"
        # ">>> Time cluster >>>"
        # ">>> Yaw >>>"
        # ">>> Stepper position >>>"
        # ">>> Encoders >>>"
        # ">>> Object detection >>>"
        # ">>> Ultrasonic Sensors Detect >>>"
        n68 = Unbundle By Name(w1235) -> ("Yaw"=w1232:dbl)
        n69 = call "MOTOR CONTROL WITH PID AE.vi"("Yaw"=w1232, "Speed"=-25.0, "Direction"=MOTOR_CONTROL_WITH_PID_AE_DIRECTION_TYPE_DEF."x-axis movement", "AE Mode"=MOTOR_CONTROL_WITH_PID_AE_DATA_MODE_TYPE_DEF."Write to AE") -> ()  [unwired: 1 out]
      }
      frame "R-ACW" {
        # ">>> IR Sensors >>>"
        # ">>> Time cluster >>>"
        # ">>> Yaw >>>"
        # ">>> Stepper position >>>"
        # ">>> Encoders >>>"
        # ">>> Object detection >>>"
        # ">>> Ultrasonic Sensors Detect >>>"
        n70 = call "MOTOR CONTROL WITH PID AE.vi"("Speed"=80.0, "Direction"=MOTOR_CONTROL_WITH_PID_AE_DIRECTION_TYPE_DEF."rotation", "AE Mode"=MOTOR_CONTROL_WITH_PID_AE_DATA_MODE_TYPE_DEF."Write to AE") -> ()  [unwired: 1 in, 1 out]
      }
      frame "R-CW" {
        (unwired) -0.2 ("Speed")
        # ">>> Time cluster >>>"
        # ">>> Yaw >>>"
        # ">>> Stepper position >>>"
        # ">>> Encoders >>>"
        # ">>> Object detection >>>"
        # ">>> Ultrasonic Sensors Detect >>>"
        n71 = call "MOTOR CONTROL WITH PID AE.vi"("Speed"=60.0, "Direction"=MOTOR_CONTROL_WITH_PID_AE_DIRECTION_TYPE_DEF."rotation", "AE Mode"=MOTOR_CONTROL_WITH_PID_AE_DATA_MODE_TYPE_DEF."Write to AE") -> ()  [unwired: 1 in, 1 out]
      }
      frame "RIGHT" {
        # ">>> Time cluster >>>"
        # ">>> Yaw >>>"
        # ">>> Stepper position >>>"
        # ">>> Encoders >>>"
        # ">>> Object detection >>>"
        # ">>> Ultrasonic Sensors Detect >>>"
        n72 = Unbundle By Name(w1269) -> ("Yaw"=w1265:dbl)
        n73 = call "MOTOR CONTROL WITH PID AE.vi"("Yaw"=w1265, "Speed"=50.0, "Direction"=MOTOR_CONTROL_WITH_PID_AE_DIRECTION_TYPE_DEF."x-axis movement", "AE Mode"=MOTOR_CONTROL_WITH_PID_AE_DATA_MODE_TYPE_DEF."Write to AE") -> ()  [unwired: 1 out]
      }
      frame "REVERSE" {
        # ">>> Time cluster >>>"
        # ">>> Yaw >>>"
        # ">>> Stepper position >>>"
        # ">>> Encoders >>>"
        # ">>> Object detection >>>"
        # ">>> Ultrasonic Sensors Detect >>>"
        n74 = Unbundle By Name(w1281) -> ("Yaw"=w1277:dbl)
        n75 = call "MOTOR CONTROL WITH PID AE.vi"("Yaw"=w1277, "Speed"=-50.0, "Direction"=MOTOR_CONTROL_WITH_PID_AE_DIRECTION_TYPE_DEF."y-axis movement", "AE Mode"=MOTOR_CONTROL_WITH_PID_AE_DATA_MODE_TYPE_DEF."Write to AE") -> ()  [unwired: 1 out]
      }
      frame "STOP" {
        n76 = Wait (ms)(milliseconds to wait=u32 100) -> ()  [unwired: 1 out]
        n77 = call "MOTOR CONTROL WITH PID AE.vi"("Direction"=MOTOR_CONTROL_WITH_PID_AE_DIRECTION_TYPE_DEF."stop", "AE Mode"=MOTOR_CONTROL_WITH_PID_AE_DATA_MODE_TYPE_DEF."Write to AE") -> ()  [unwired: 2 in, 1 out]
      }
      frame "----SENSOR READING---- " {
      }
      frame "READ ENCODERS" {
        # ">>> Time cluster >>>"
        # ">>> Yaw >>>"
        # ">>> Stepper position >>>"
        # ">>> Object detection >>>"
        # ">>> Current encoder distance >>>"
        # ">>> Ultrasonic Sensors Detect >>>"
        n78 = call "MOTOR CONTROL WITH PID AE.vi"("AE Mode"=MOTOR_CONTROL_WITH_PID_AE_DATA_MODE_TYPE_DEF."Read from AE") -> ("Speed & distance"=w1311:T1)  [unwired: 3 in]
        n79 = Unbundle By Name(w1311) -> ("xDistance"=w1310:dbl, "yDistance"=w1309:dbl, "wDistance"=w1308:dbl)
        n80 = Bundle By Name(cluster=w1318, "xDistance"=w1310, "yDistance"=w1309, "wDistance"=w1308) -> (w1317:T16)
      }
      frame "READ ULTRASONIC" {
        (unwired) navX_type_def."Read Values" ("Mode")
        (unwired) MOTOR_CONTROL_NO_PID_Type_Def."Latch" ("Direction")
        # ">>State Logic  >>"
        # ">>> Time cluster >>>"
        # ">>> Ultrasonic Sensors Detect >>>"
        # ">>> Object detection >>>"
        # ">>> Encoders >>>"
        # ">>> Stepper position >>>"
        # ">>> Yaw >>>"
        n81 = call "Arduino Interfacing VI.vi"("AE Mode"=Arduino_Interfacing."Read From Arduino") -> ("Arduino Data"=w1328:T4)  [unwired: 3 in, 1 out]
        n82 = Unbundle By Name(w1328) -> ("PING A"=w1327:u8, "PING B"=w1326:u8, "PING C"=w1325:u8, "PING D"=w1324:u8)
        n83 = Bundle By Name(cluster=w1334, "PING_A"=w1327, "PING_B"=w1326, "PING_C"=w1325, "PING_D"=w1324) -> (w1335:T15)
      }
      frame "READ NAVX" {
        # ">>> Time cluster >>>"
        # ">>> Yaw >>>"
        # ">>> Ultrasonic Sensors Detect >>>"
        # ">>> Object detection >>>"
        # ">>> Encoders >>>"
        # ">>> Stepper position >>>"
        n84 = call "navX reading VI.vi"("Mode"=navX_type_def."Read Values") -> ("NavX Readings"=w1338:T3)  [unwired: 2 in, 3 out]
        n85 = Unbundle By Name(w1338) -> ("Heading"=w1337:dbl)
        n86 = Unbundle By Name(w1338) -> ("Yaw"=w1341:dbl)
        n87 = Bundle By Name(cluster=w1343, "Yaw"=w1341, "Compass"=w1337) -> (w1342:T11)
      }
      frame "READ IR" {
        w1353 = T33 [enum."A/AI0"] items=["Not Connected", "AudioIn/Left", "AudioIn/Right", "C/AI0", "C/AI1", "A/AI0", "A/AI1", "A/AI2", "A/AI3", "A/AI4", "A/AI5", "A/AI6", "A/AI7", "B/AI0", "B/AI1", "B/AI2", "B/AI3", "B/AI4", "B/AI5", "B/AI6", "B/AI7", "AI/AI0", "AI/AI1", "AI/AI2", "AI/AI3", "A/AI0 (DIFF)", "A/AI1 (DIFF)", "A/AI2 (DIFF)", "A/AI3 (DIFF)", "B/AI0 (DIFF)", "B/AI1 (DIFF)", "B/AI2 (DIFF)", "B/AI3 (DIFF)"] ("AI Channel")
        # ">>State Logic  >>"
        # ">>> Time cluster >>>"
        # ">>> Ultrasonic Sensors Detect >>>"
        # ">>> Object detection >>>"
        # ">>> Encoders >>>"
        # ">>> Stepper position >>>"
        # ">>> Yaw >>>"
        n88 = call <vilib>:"Sharp IR.vi"("AI Channel"=w1353) -> ("Sharp IR Distance"=w1349:dbl)  [unwired: 8 in, 2 out]
        n89 = Bundle By Name(cluster=w1351, "Left IR Sensor"=w1349) -> (w1350:T8)
      }
      frame "----SYSTEM MODES----" {
        (unwired) I2C_MASTER_Type_Def."Last State" ("Arduino Mode")
        # ">>> Object detection >>>"
        # ">>> Yaw >>>"
        # ">>> Ultrasonic Sensors Detect >>>"
        # ">>> Encoders >>>"
        # ">>> Stepper position >>>"
      }
      frame "INIT" {
        w1386 = u8 0
        w1387 = 0.0
        # ">>> Time cluster >>>"
        # ">>> Object detection >>>"
        # ">>> Yaw >>>"
        # ">>> Ultrasonic Sensors Detect >>>"
        # ">>> Encoders >>>"
        # ">>> Stepper position >>>"
        # ">>State Logic  >>"
        n90 = call "Arduino Interfacing VI.vi"("AE Mode"=Arduino_Interfacing."Initialize") -> ()  [unwired: 3 in, 2 out]
        n91 = call "FGV Bool.vi"("Init/Read/Write State"=States_for_Action_Engine."Initialize") -> ()  [unwired: 2 in, 2 out]
        n92 = call "Elasped Timer.vi"("Action"=Elapsed_timer_control."Initialize") -> ()  [unwired: 7 in, 4 out]
        n93 = call "MOTOR CONTROL WITH PID AE.vi"("AE Mode"=MOTOR_CONTROL_WITH_PID_AE_DATA_MODE_TYPE_DEF."Init AE") -> ()  [unwired: 3 in, 1 out]
        n94 = Bundle By Name(cluster=w1380, "Recognized Object"=FALSE, "Object X coordinate"=0.0, "Object Y coordinate"=0.0) -> (w1379:T14)
        n95 = Bundle By Name(cluster=w1385, "y Stepper Position"=u8 0, "z Stepper Position"=u8 0) -> (w1384:T12)
        n96 = Bundle By Name(cluster=w1389, "xDistance"=w1387, "yDistance"=w1387, "wDistance"=w1387) -> (w1388:T16)
        n97 = Bundle By Name(cluster=w1391, "PING_A"=w1386, "PING_B"=w1386, "PING_C"=w1386, "PING_D"=w1386) -> (w1392:T15)
        n98 = Bundle By Name(cluster=w1375, "Yaw"=0.0) -> (w1374:T11)
      }
      frame "ARDUINO - ULTRASONIC" {
        # ">>> Object detection >>>"
        # ">>> Yaw >>>"
        # ">>> Ultrasonic Sensors Detect >>>"
        # ">>> Encoders >>>"
        # ">>> Stepper position >>>"
        # ">>State Logic  >>"
        n99 = call "Arduino Interfacing VI.vi"("Data to Write"=I2C_MASTER_WRITE_NEW_Type_Def."Ultrasonic sensors", "AE Mode"=Arduino_Interfacing."Write to Arduino") -> ()  [unwired: 2 in, 2 out]
      }
      frame "NAVX CALIBRATE" {
        # ">>> Object detection >>>"
        # ">>> Yaw >>>"
        # ">>> Ultrasonic Sensors Detect >>>"
        # ">>> Encoders >>>"
        # ">>> Stepper position >>>"
        # ">>State Logic  >>"
        # "Adds a 15 second delay to the startup process \nfor the NavX to calibrate"
        n100 = Wait (ms)(milliseconds to wait=u32 5000) -> ()  [unwired: 1 out]
      }
      frame "NO ACTION", Default {
        (unwired) u8 0 ("y Stepper value")
        (unwired) TRUE ("Latch")
        (unwired) navX_type_def."Read Values" ("Mode")
        (unwired) MOTOR_CONTROL_NO_PID_Type_Def."Latch" ("Direction")
        # ">>> Object detection >>>"
        # ">>> Yaw >>>"
        # ">>> Ultrasonic Sensors Detect >>>"
        # ">>> Encoders >>>"
        # ">>> Stepper position >>>"
        # ">>State Logic  >>"
        n101 = case shown="4" w1419 {
          tunnel: [0 100] -> w1421
          frame 1, Default {
          }
          frame 4 {
          }
        }
      }
      frame "----RESET CASES----" {
        (unwired) I2C_MASTER_Type_Def."Last State" ("Arduino Mode")
        # ">>> Object detection >>>"
        # ">>> Yaw >>>"
        # ">>> Ultrasonic Sensors Detect >>>"
        # ">>> Encoders >>>"
        # ">>> Stepper position >>>"
        # ">>State Logic  >>"
      }
      frame "RESET ENCODERS" {
        # ">>> Object detection >>>"
        # ">>> Yaw >>>"
        # ">>> Ultrasonic Sensors Detect >>>"
        # ">>> Encoders >>>"
        # ">>> Stepper position >>>"
        # ">>State Logic  >>"
        n102 = call "MOTOR CONTROL WITH PID AE.vi"("Direction"=MOTOR_CONTROL_WITH_PID_AE_DIRECTION_TYPE_DEF."reset encoders", "AE Mode"=MOTOR_CONTROL_WITH_PID_AE_DATA_MODE_TYPE_DEF."Write to AE") -> ()  [unwired: 2 in, 1 out]
      }
      frame "RESET FLAGS" {
        (unwired) I2C_MASTER_Type_Def."Last State" ("Arduino Mode")
        # "Resets any software variables\nand/or non-critical states"
        n103 = Wait (ms)(milliseconds to wait=u32 20) -> ()  [unwired: 1 out]
        n104 = Bundle By Name(cluster=w1447, "Time up flag"=FALSE, "SET TIME TO CHECK"=0.0) -> (w1446:T10)
        n105 = Bundle By Name(cluster=w1464, "Recognized Object"=FALSE, "Object X coordinate"=0.0, "Object Y coordinate"=0.0) -> (w1463:T14)
        n106 = Bundle By Name(cluster=w1454, "y Stepper Position"=u8 0, "z Stepper Position"=u8 0) -> (w1453:T12)
        n107 = Bundle By Name(cluster=w1459, "xDistance"=0.0, "yDistance"=0.0, "wDistance"=0.0) -> (w1458:T16)
        n108 = Bundle By Name(cluster=w1471, "PING_A"=u8 0, "PING_B"=u8 0, "PING_C"=u8 0, "PING_D"=u8 0) -> (w1470:T15)
        n109 = Bundle By Name(cluster=w1450, "Yaw"=0.0) -> (w1449:T11)
      }
      frame "RESET YAW" {
        n110 = Wait (ms)(milliseconds to wait=u32 100) -> ()  [unwired: 1 out]
        n111 = call "navX reading VI.vi"("Mode"=navX_type_def."Zero Yaw") -> ()  [unwired: 2 in, 4 out]
      }
      frame "RESET ARM" {
        n112 = call "Arduino Interfacing VI.vi"("Data to Write"=I2C_MASTER_WRITE_NEW_Type_Def."Soft Reset", "AE Mode"=Arduino_Interfacing."Write to Arduino") -> ()  [unwired: 2 in, 2 out]
      }
      frame "--------CAM STATES-------" {
      }
      frame "OPEN LOG CAM" {
        n113 = call "Webcam AE.vi"("Session In"=T30 "cam0", "Camera states"=Webcam_AE."Initialize Camera") -> ("error out"=w1504:errorcluster, "Session Out"=w1503:T30)  [unwired: 1 in, 1 out]
        n114 = call "Webcam AE.vi"("error in (no error)"=w1504, "Session In"=w1503, "Camera states"=Webcam_AE."Open Camera") -> ()  [unwired: 3 out]
      }
      frame "OPEN LIFE CAM" {
        n115 = call "Webcam AE.vi"("Session In"=T30 "cam1", "Camera states"=Webcam_AE."Initialize Camera") -> ("error out"=w1517:errorcluster, "Session Out"=w1516:T30)  [unwired: 1 in, 1 out]
        n116 = call "Webcam AE.vi"("error in (no error)"=w1517, "Session In"=w1516, "Camera states"=Webcam_AE."Open Camera") -> ()  [unwired: 3 out]
      }
      frame "CAM ACQ" {
        # ">>State Logic  >>"
        # ">>> Time cluster >>>"
        # ">>> Yaw >>>"
        # ">>> Stepper position >>>"
        # ">>> Encoders >>>"
        # ">>> Object detection >>>"
        # ">>> Ultrasonic Sensors Detect >>>"
        n117 = call "Webcam AE.vi"("error in (no error)"=w1528, "Camera states"=Webcam_AE."Continuous Acquisition") -> ()  [unwired: 1 in, 3 out]
      }
      frame "CAM CLOSE" {
        # ">>State Logic  >>"
        # ">>> Time cluster >>>"
        # ">>> Yaw >>>"
        # ">>> Stepper position >>>"
        # ">>> Encoders >>>"
        # ">>> Object detection >>>"
        # ">>> Ultrasonic Sensors Detect >>>"
        n118 = call "Webcam AE.vi"("Camera states"=Webcam_AE."Close Camera") -> ()  [unwired: 2 in, 3 out]
      }
      frame "PROCESS IMAGE" {
        # ">>State Logic  >>"
        # ">>> Time cluster >>>"
        # ">>> Yaw >>>"
        # ">>> Stepper position >>>"
        # ">>> Encoders >>>"
        # ">>> Object detection >>>"
        # ">>> Ultrasonic Sensors Detect >>>"
        n119 = call "Webcam AE.vi"("error in (no error)"=w1558, "Camera states"=Webcam_AE."Retrieve Image") -> ("error out"=w1554:errorcluster, "Image Out"=w1557:T23)  [unwired: 1 in, 1 out]
        n120 = call "Object Detection SubVI.vi"("Error In"=w1554, "Mode"="Object recognition mode", "Image Dest"=w1556, "Image in"=w1557) -> ("Object Center Coordinates"=w1551:cluster{"x":sgl, "y":sgl}, "Object detection cluster"=w1547:T2)  [unwired: 2 out]
        "Object detection cluster" <- w1547
        "Object Center Coordinates" <- w1551
        n121 = Unbundle By Name(w1547) -> ("Object detected?"=w1548:bool)
        n122 = Unbundle By Name(w1551) -> ("x"=w1550:sgl, "y"=w1549:sgl)
        n123 = Bundle By Name(cluster=w1553, "Recognized Object"=w1548, "Object X coordinate"=w1550, "Object Y coordinate"=w1549) -> (w1552:T14)
      }
      frame "DISPOSE BUFFERS" {
        # ">>State Logic  >>"
        # ">>> Time cluster >>>"
        # ">>> Yaw >>>"
        # ">>> Stepper position >>>"
        # ">>> Encoders >>>"
        # ">>> Object detection >>>"
        # ">>> Ultrasonic Sensors Detect >>>"
        n124 = call "Webcam AE.vi"("error in (no error)"=w1568, "Camera states"=Webcam_AE."Dispose Image Buffers") -> ()  [unwired: 1 in, 3 out]
      }
      frame "-----ARM ACTIONS-----" {
      }
      frame "CLOSE CLAW" {
        n125 = call "Arduino Interfacing VI.vi"("Data to Write"=I2C_MASTER_WRITE_NEW_Type_Def."Close Claw", "AE Mode"=Arduino_Interfacing."Write to Arduino") -> ()  [unwired: 2 in, 2 out]
      }
      frame "OPEN CLAW" {
        n126 = call "Arduino Interfacing VI.vi"("Data to Write"=I2C_MASTER_WRITE_NEW_Type_Def."Open Claw", "AE Mode"=Arduino_Interfacing."Write to Arduino") -> ()  [unwired: 2 in, 2 out]
      }
      frame "Z STEPPER CAM HEIGHT" {
        n127 = call "Arduino Interfacing VI.vi"("Data to Write"=I2C_MASTER_WRITE_NEW_Type_Def."zStepper 8k", "AE Mode"=Arduino_Interfacing."Write to Arduino") -> ()  [unwired: 2 in, 2 out]
      }
      frame "Z STEPPER GRAB HEIGHT" {
        # ">>State Logic  >>"
        # ">>> Time cluster >>>"
        # ">>> Yaw >>>"
        # ">>> Stepper position >>>"
        # ">>> Encoders >>>"
        # ">>> Object detection >>>"
        # ">>> Ultrasonic Sensors Detect >>>"
        n128 = call "Arduino Interfacing VI.vi"("Data to Write"=I2C_MASTER_WRITE_NEW_Type_Def."zStepper 100", "AE Mode"=Arduino_Interfacing."Write to Arduino") -> ()  [unwired: 2 in, 2 out]
      }
      frame "Y STEPPER CONTROL" {
        # ">>State Logic  >>"
        # ">>> yStepper command>>>"
        # ">>> Time cluster >>>"
        # ">>> Yaw >>>"
        # ">>> Stepper position >>>"
        # ">>> Encoders >>>"
        # ">>> Object detection >>>"
        # ">>> Ultrasonic Sensors Detect >>>"
        n129 = Unbundle By Name(w1626) -> ("yStepper desired"=w1625:u8)
        n130 = call "Arduino Interfacing VI.vi"("y Stepper value"=w1625, "Data to Write"=I2C_MASTER_WRITE_NEW_Type_Def."yStepper control", "AE Mode"=Arduino_Interfacing."Write to Arduino") -> ()  [unwired: 1 in, 2 out]
      }
      frame "READ STEPPER VALUES" {
        # ">>State Logic  >>"
        # ">>> Time cluster >>>"
        # ">>> Yaw >>>"
        # ">>> Stepper position >>>"
        # ">>> Encoders >>>"
        # ">>> Object detection >>>"
        # ">>> Ultrasonic Sensors Detect >>>"
        n131 = call "Arduino Interfacing VI.vi"("AE Mode"=Arduino_Interfacing."Read From Arduino") -> ("Arduino Data"=w1641:T4)  [unwired: 3 in, 1 out]
        n132 = Unbundle By Name(w1641) -> ("y Stepper Position"=w1640:u8, "z Stepper Position"=w1639:u8)
        n133 = Bundle By Name(cluster=w1644, "y Stepper Position"=w1640, "z Stepper Position"=w1639) -> (w1643:T12)
      }
      frame " -----TIMING-----" {
        # ">>State Logic  >>"
        # ">>> Time cluster >>>"
        # ">>> Yaw >>>"
        # ">>> Stepper position >>>"
        # ">>> Encoders >>>"
        # ">>> Object detection >>>"
        # ">>> Ultrasonic Sensors Detect >>>"
      }
      frame "SET TIMER 1" {
        # ">>State Logic  >>"
        # ">>> Time cluster >>>"
        # ">>> Yaw >>>"
        # ">>> Stepper position >>>"
        # ">>> Encoders >>>"
        # ">>> Object detection >>>"
        # ">>> Ultrasonic Sensors Detect >>>"
        n134 = call "Elasped Timer.vi"("Time Setting"=1.0, "Action"=Elapsed_timer_control."Initialize") -> ()  [unwired: 6 in, 4 out]
        n135 = Bundle By Name(cluster=w1662, "Time up flag"=FALSE) -> (w1660:T10)
      }
      frame "SET TIMER 2" {
        # ">>State Logic  >>"
        # ">>> Time cluster >>>"
        # ">>> Yaw >>>"
        # ">>> Stepper position >>>"
        # ">>> Encoders >>>"
        # ">>> Object detection >>>"
        # ">>> Ultrasonic Sensors Detect >>>"
        n136 = call "Elasped Timer.vi"("Time Setting"=2.0, "Action"=Elapsed_timer_control."Initialize") -> ()  [unwired: 6 in, 4 out]
        n137 = Bundle By Name(cluster=w1674, "Time up flag"=FALSE) -> (w1672:T10)
      }
      frame "SET TIMER 3" {
        # ">>State Logic  >>"
        # ">>> Time cluster >>>"
        # ">>> Yaw >>>"
        # ">>> Stepper position >>>"
        # ">>> Encoders >>>"
        # ">>> Object detection >>>"
        # ">>> Ultrasonic Sensors Detect >>>"
        n138 = call "Elasped Timer.vi"("Time Setting"=3.0, "Action"=Elapsed_timer_control."Initialize") -> ()  [unwired: 6 in, 4 out]
        n139 = Bundle By Name(cluster=w1686, "Time up flag"=FALSE) -> (w1684:T10)
      }
      frame "SET TIMER 4" {
        # ">>State Logic  >>"
        # ">>> Time cluster >>>"
        # ">>> Yaw >>>"
        # ">>> Stepper position >>>"
        # ">>> Encoders >>>"
        # ">>> Object detection >>>"
        # ">>> Ultrasonic Sensors Detect >>>"
        n140 = call "Elasped Timer.vi"("Time Setting"=4.0, "Action"=Elapsed_timer_control."Initialize") -> ()  [unwired: 6 in, 4 out]
        n141 = Bundle By Name(cluster=w1698, "Time up flag"=FALSE) -> (w1696:T10)
      }
      frame "SET TIMER 5" {
        # ">>State Logic  >>"
        # ">>> Time cluster >>>"
        # ">>> Yaw >>>"
        # ">>> Stepper position >>>"
        # ">>> Encoders >>>"
        # ">>> Object detection >>>"
        # ">>> Ultrasonic Sensors Detect >>>"
        n142 = call "Elasped Timer.vi"("Time Setting"=5.0, "Action"=Elapsed_timer_control."Initialize") -> ()  [unwired: 6 in, 4 out]
        n143 = Bundle By Name(cluster=w1710, "Time up flag"=FALSE) -> (w1708:T10)
      }
      frame "START TIMER" {
        # ">>State Logic  >>"
        # ">>> Time cluster >>>"
        # ">>> Yaw >>>"
        # ">>> Stepper position >>>"
        # ">>> Encoders >>>"
        # ">>> Object detection >>>"
        # ">>> Ultrasonic Sensors Detect >>>"
        n144 = call "Elasped Timer.vi"("Action"=Elapsed_timer_control."Start") -> ("Time Out?!"=w1718:bool)  [unwired: 7 in, 3 out]
        n145 = Bundle By Name(cluster=w1721, "Time up flag"=w1718) -> (w1720:T10)
      }
    }
    "State Logic" <- w225
    n146 = local read "TASK ENABLE"() -> (w219:bool)
    n147 = Not(x=w219) -> (.not. x?=w218:bool)
    n148 = case shown="True" w226 {
      tunnel: w230 -> [w254 w287]
      tunnel: w234 -> [w250 w289]
      tunnel: [w254 w287] -> w239
      tunnel: [w250 w290] -> w238
      tunnel: w235 -> [_ w285]
      tunnel: w237 -> [_ w286]
      tunnel: w232 -> [w253 w292]
      tunnel: [w253 w292] -> w231
      tunnel: "STOP TASK" -> [_ w275]
      tunnel: w225 -> [w252 w291]
      tunnel: [w252 w288] -> w224
      tunnel: w221 -> [w251 w281]
      tunnel: [w251 w281] -> w220
      tunnel: w218 -> [_ w276]
      tunnel: [w249 w273] -> w217
      tunnel: w216 -> [w249 w272]
      tunnel: w212 -> [w248 w269]
      tunnel: [w248 w269] -> w211
      tunnel: w209 -> [w247 w265]
      tunnel: [w247 w265] -> w208
      tunnel: w206 -> [w246 w263]
      tunnel: [w246 w263] -> w205
      tunnel: w203 -> [w245 w261]
      tunnel: [w245 w261] -> w202
      tunnel: w201 -> [w244 w260]
      tunnel: [w244 w259] -> w200
      tunnel: [_ w257] -> w199
      tunnel: w197 -> [w243 w255]
      tunnel: [w243 w255] -> w196
      frame False {
        # ">>> IR Sensors >>>"
        # ">>> IR Sensors >>>"
        # ">>> yStepper command>>>"
        # ">>> Time cluster >>>"
        # ">>> Yaw >>>"
        # ">>> Stepper position >>>"
        # ">>> Encoders >>>"
        # ">>> Object detection >>>"
        # ">>> Ultrasonic Sensors Detect >>>"
        # ">>> Time cluster >>>"
        # ">>> Yaw >>>"
        # ">>> Stepper position >>>"
        # ">>> Encoders >>>"
        # ">>> Object detection >>>"
        # ">>> Ultrasonic Sensors Detect >>>"
      }
      frame True {
        # ">>State Logic Queue Reference >>"
        # ">>Timeout>>"
        # ">>> yStepper command>>>"
        # ">>> Time cluster >>>"
        # ">>> Object detection >>>"
        # ">>> Yaw >>>"
        # ">>> Ultrasonic Sensors Detect >>>"
        # ">>> Encoders >>>"
        # ">>> Stepper position >>>"
        # ">>State Logic  >>"
        # ">>True Stop Next State >>"
        # ">>Action Queue>>"
        # ">> Manual override >>"
        # ">>> Time cluster >>>"
        # ">>> Yaw >>>"
        # ">>> Stepper position >>>"
        # ">>> Encoders >>>"
        # ">>> Object detection >>>"
        # ">>> Ultrasonic Sensors Detect >>>"
        # ">>Action Queue>>"
        # ">>State Logic Queue Reference >>"
        n149 = Or(x=w275, y=w276) -> (x .or. y?=w274:bool)
        n150 = Unbundle By Name(w255) -> ("Left IR Sensor"=w256:dbl)
        "Left IR Sensor" <- w256
        n151 = Unbundle By Name(w261) -> ("Time up flag"=w262:bool)
        "Time up flag" <- w262
        n152 = Unbundle By Name(w263) -> ("Yaw"=w264:dbl, "Compass"=w258:dbl)
        n153 = Unbundle By Name(w265) -> ("y Stepper Position"=w267:u8, "z Stepper Position"=w266:u8)
        n154 = Unbundle By Name(w281) -> ("xDistance"=w278:dbl, "yDistance"=w279:dbl, "wDistance"=w280:dbl)
        n155 = Unbundle By Name(w269) -> ("Recognized Object"=w268:bool, "Object X coordinate"=w271:dbl, "Object Y coordinate"=w270:dbl)
        n156 = Unbundle By Name(w292) -> ("PING_A"=w284:u8, "PING_B"=w283:u8, "PING_C"=w282:u8, "PING_D"=w277:u8)
        n157 = case shown="9" w291 {
          tunnel: [w295 w301 w313 w322 w389 w402 w437 w489 w528 w574 w616 w669 w715 w754 w813 w857 w896 w941 w984 w1026 w1056 w1103 w1143] -> w290
          tunnel: w289 -> [w295 w304 w314 w325 w391 w403 w446 w487 w532 w575 w622 w662 w718 w761 w803 w860 w902 w940 w979 w1017 w1060 w1110 w1148]
          tunnel: [State_Type_Definitions."Idle" ("Enum") State_Type_Definitions."Idle" ("Enum") w309 w324 State_Type_Definitions."Shutdown" ("Enum") w404 w444 w490 w529 w573 w617 w668 w716 w756 w812 w858 w903 w942 w985 w1018 w1057 w1104 w1144] -> w288
          tunnel: w287 -> [_ _ w312 w328 _ w409 w440 w486 w533 w582 w621 w666 w719 w760 w810 w855 w901 w938 w982 w1025 w1064 w1109 w1151]
          tunnel: w286 -> [_ _ _ w327 _ w408 w439 w485 w534 w581 w620 w665 w712 w759 w809 w854 w900 w937 w981 w1023 w1059 w1108 w1150]
          tunnel: w285 -> [_ _ w311 w323 _ w407 w438 w484 w535 w580 w619 w664 w711 w758 w811 w856 w899 w936 w980 w1024 w1063 w1107 w1149]
          tunnel: w274 -> [_ _ _ _ _ w401 w445 w483 w536 w577 w615 w667 w717 w762 w804 w861 w897 w939 w983 w1021 w1062 w1102 w1147]
          tunnel: w284 -> [_ _ _ _ _ _ _ _ _ _ _ _ _ _ _ _ _ _ _ _ _ _ _]
          tunnel: w283 -> [_ _ _ _ _ _ _ w482 _ _ _ w658 w700 w752 _ w847 _ _ _ _ _ _ _]
          tunnel: w282 -> [_ _ _ _ _ _ _ w481 _ _ _ w659 w701 w753 _ w848 _ _ _ _ _ _ _]
          tunnel: w280 -> [_ _ _ _ _ _ _ _ _ w579 _ _ _ _ _ _ _ _ _ _ _ _ _]
          tunnel: w279 -> [_ _ _ _ _ w400 _ _ _ _ _ _ _ w757 _ _ _ _ _ _ _ _ _]
          tunnel: w278 -> [_ _ _ _ _ _ _ _ _ _ _ _ w706 _ _ _ _ _ _ _ _ _ _]
          tunnel: w277 -> [_ _ _ _ _ _ _ _ _ _ _ _ _ _ _ _ _ _ _ _ _ _ _]
          tunnel: [State_Type_Definitions."Idle" ("Enum") State_Type_Definitions."Idle" ("Enum") State_Type_Definitions."Idle" ("Enum") State_Type_Definitions."Idle" ("Enum") State_Type_Definitions."Shutdown" ("Enum") w397 w443 w488 w530 w570 w614 w661 w714 w755 w814 w859 w895 w943 w986 w1019 w1058 w1105 w1146] -> w273
          tunnel: w272 -> [_ _ w309 _ _ _ _ _ _ _ _ _ _ _ _ _ _ _ _ _ _ _ _]
          tunnel: w268 -> [_ _ _ _ _ _ _ _ _ _ _ _ _ _ _ _ _ w933 _ w1020 _ _ _]
          tunnel: w271 -> [_ _ _ _ _ _ _ _ _ _ _ _ _ _ _ _ _ _ _ _ _ _ _]
          tunnel: w270 -> [_ _ _ _ _ _ _ _ _ _ _ _ _ _ _ _ _ _ _ _ _ _ _]
          tunnel: w267 -> [_ _ _ _ _ _ _ _ _ _ _ _ _ _ _ _ _ _ _ _ _ _ _]
          tunnel: w266 -> [_ _ _ _ _ _ w442 _ _ _ w612 _ _ _ w807 _ _ _ w978 _ w1061 _ _]
          tunnel: w264 -> [_ _ _ _ _ _ _ _ _ _ _ _ _ _ _ _ _ _ _ _ _ _ _]
          tunnel: w262 -> [_ _ _ _ _ _ _ _ w527 _ _ _ _ _ _ _ w893 _ _ _ _ _ _]
          tunnel: w260 -> [w293 w299 w308 w320 w387 w396 w441 w480 w531 w569 w613 w660 w710 w751 w802 w852 w894 w934 w975 w1016 w1055 w1106 w1145]
          tunnel: [w293 w298 w308 w320 w387 w396 w441 w480 w531 w569 w613 w660 w710 w751 w802 w852 w894 w934 w975 w1016 w1055 w1106 w1145] -> w259
          tunnel: w258 -> [_ _ _ _ _ _ _ _ _ _ _ _ _ _ _ _ _ _ _ _ _ w1101 _]
          tunnel: [_ _ _ TRUE _ _ _ _ _ _ _ _ _ _ _ _ _ _ _ _ _ _ _] -> w257
          tunnel: w256 -> [_ _ _ _ _ _ _ _ _ _ _ _ _ _ _ _ _ _ _ _ _ _ _]
          frame 0 {
            # ">>> yStepper command>>>"
          }
          frame 1 {
            # ">>> yStepper command>>>"
            n158 = for {
              shift-right: [w307] -> w301
              shift-left: w304 -> [w306]
              tunnel: string[] ["INIT", "RESET ARM", "RESET FLAGS", "RESET YAW", "NAVX CALIBRATE"] -> [w305] mode=indexing
              n159 = Enqueue Element(queue=w306, element=w305) -> (queue out=w307:refnum<queue>)  [unwired: 2 in, 2 out]
            }
            n160 = Bundle By Name(cluster=w299, "yStepper desired"=u8 0) -> (w298:T9)
          }
          frame 3 {
            # ">>> yStepper command>>>"
            n161 = Flush Queue(queue=w312, error in (no error)=w311) -> ()  [unwired: 3 out]
            n162 = for {
              shift-right: [w318] -> w313
              shift-left: w314 -> [w317]
              tunnel: string[] ["STOP", "RESET ENCODERS", "RESET YAW", "RESET ARM", "RESET FLAGS", "DISPOSE BUFFERS", "CAM CLOSE"] -> [w316] mode=indexing
              n163 = Enqueue Element(queue=w317, element=w316) -> (queue out=w318:refnum<queue>)  [unwired: 2 in, 2 out]
            }
          }
          frame 4, Default {
            (unwired) TRUE ("Green LED")
            # ">>> yStepper command>>>"
            n164 = Dequeue Element(queue=w328, timeout in ms (-1)=w327, error in (no error)=w323) -> (element=w326:T7)  [unwired: 3 out]
            n165 = case shown="\"Start Task 9\"" w326 {
              tunnel: [w330 w337 w344 w351 w358 w365 w372 w374 w382] -> w322
              tunnel: w325 -> [w331 w338 w345 w352 w359 w366 w372 w375 w381]
              tunnel: [State_Type_Definitions."Task 1" ("Enum") State_Type_Definitions."Task 2:Raise Arm" ("Enum") State_Type_Definitions."Task 3" ("Enum") State_Type_Definitions."Task 4_A" ("Enum") State_Type_Definitions."Task 5_A" ("Enum") State_Type_Definitions."Task 6_A" ("Enum") State_Type_Definitions."Idle" ("Enum") State_Type_Definitions."Shutdown" ("Enum") State_Type_Definitions."Task 9A: Raise Arm" ("Enum")] -> w324
              frame "Start Task 1" {
                n166 = for {
                  shift-right: [w335] -> w330
                  shift-left: w331 -> [w334]
                  tunnel: string[] ["RESET ENCODERS", "RESET YAW", "FORWARD", "READ ENCODERS"] -> [w333] mode=indexing
                  n167 = Enqueue Element(queue=w334, element=w333) -> (queue out=w335:refnum<queue>)  [unwired: 2 in, 2 out]
                }
              }
              frame "Start Task 2" {
                n168 = for {
                  shift-right: [w342] -> w337
                  shift-left: w338 -> [w341]
                  tunnel: string[] ["RESET ENCODERS", "RESET YAW", "READ ULTRASONIC", "ARDUINO - ULTRASONIC"] -> [w340] mode=indexing
                  n169 = Enqueue Element(queue=w341, element=w340) -> (queue out=w342:refnum<queue>)  [unwired: 2 in, 2 out]
                }
              }
              frame "Start Task 3" {
                n170 = for {
                  shift-right: [w349] -> w344
                  shift-left: w345 -> [w348]
                  tunnel: string[] ["RESET ENCODERS", "READ ENCODERS", "R-ACW"] -> [w347] mode=indexing
                  n171 = Enqueue Element(queue=w348, element=w347) -> (queue out=w349:refnum<queue>)  [unwired: 2 in, 2 out]
                }
              }
              frame "Start Task 4" {
                n172 = for {
                  shift-right: [w356] -> w351
                  shift-left: w352 -> [w355]
                  tunnel: string[] ["RESET YAW", "RESET ENCODERS", "RESET ARM", "RESET FLAGS", "", ""] -> [w354] mode=indexing
                  n173 = Enqueue Element(queue=w355, element=w354) -> (queue out=w356:refnum<queue>)  [unwired: 2 in, 2 out]
                }
              }
              frame "Start Task 5" {
                n174 = for {
                  shift-right: [w363] -> w358
                  shift-left: w359 -> [w362]
                  tunnel: string[] ["RESET YAW", "RESET ENCODERS", "READ STEPPER VALUES", "Z STEPPER CAM HEIGHT", "", ""] -> [w361] mode=indexing
                  n175 = Enqueue Element(queue=w362, element=w361) -> (queue out=w363:refnum<queue>)  [unwired: 2 in, 2 out]
                }
              }
              frame "Start Task 6" {
                n176 = for {
                  shift-right: [w370] -> w365
                  shift-left: w366 -> [w369]
                  tunnel: string[] ["OPEN LOG CAM ", "", "", "", "", ""] -> [w368] mode=indexing
                  n177 = Enqueue Element(queue=w369, element=w368) -> (queue out=w370:refnum<queue>)  [unwired: 2 in, 2 out]
                }
              }
              frame "None", Default {
              }
              frame "Exit" {
                n178 = for {
                  shift-right: [w379] -> w374
                  shift-left: w375 -> [w378]
                  tunnel: string[] ["STOP", "RESET ENCODERS", "RESET YAW", "EXIT"] -> [w377] mode=indexing
                  n179 = Enqueue Element(queue=w378, element=w377) -> (queue out=w379:refnum<queue>)  [unwired: 2 in, 2 out]
                }
              }
              frame "Start Task 9" {
                n180 = for {
                  shift-right: [w386] -> w382
                  shift-left: w381 -> [w385]
                  tunnel: string[] ["RESET ENCODERS", "READ ENCODERS", "Z STEPPER CAM HEIGHT"] -> [w384] mode=indexing
                  n181 = Enqueue Element(queue=w385, element=w384) -> (queue out=w386:refnum<queue>)  [unwired: 2 in, 2 out]
                }
              }
            }
          }
          frame 5 {
            # ">>> yStepper command>>>"
            n182 = for {
              shift-right: [w395] -> w389
              shift-left: w391 -> [w394]
              tunnel: string[] ["INIT", "RESET ENCODERS", "RESET FLAGS", "CAM CLOSE", "DISPOSE BUFFERS", "EXIT", ""] -> [w393] mode=indexing
              n183 = Enqueue Element(queue=w394, element=w393) -> (queue out=w395:refnum<queue>)  [unwired: 2 in, 2 out]
            }
          }
          frame 6 {
            # ">>> yStepper command>>>"
            # "Use 250"
            n184 = Dequeue Element(queue=w409, timeout in ms (-1)=w408, error in (no error)=w407) -> (element=w406:T7)  [unwired: 3 out]
            n185 = Greater?(x=w400, y=265.0) -> (0:w398:bool)
            n186 = Or(x=w398, y=w401) -> (x .or. y?=w405:bool)
            n187 = case shown="\"None\", Default" w406 {
              tunnel: w405 -> [w412 _]
              tunnel: [w416 State_Type_Definitions."True Stop" ("Enum")] -> w404
              tunnel: w403 -> [w413 w431]
              tunnel: [w411 w430] -> w402
              tunnel: [State_Type_Definitions."Idle" ("Enum") State_Type_Definitions."Shutdown" ("Enum")] -> w397
              frame "None", Default {
                n188 = case shown="True" w412 {
                  tunnel: w413 -> [w419 w425]
                  tunnel: [w418 w423] -> w411
                  frame False {
                    n189 = for {
                      shift-right: [w421] -> w418
                      shift-left: w419 -> [w422]
                      tunnel: string[] ["READ ENCODERS", "READ NAVX", "FORWARD"] ("element") -> [w420] mode=indexing
                      n190 = Enqueue Element(queue=w422, element=w420) -> (queue out=w421:refnum<queue>)  [unwired: 2 in, 2 out]
                    }
                  }
                  frame True {
                    n191 = for {
                      shift-right: [w427] -> w423
                      shift-left: w425 -> [w428]
                      tunnel: string[] ["RESET YAW", "RESET ENCODERS", "STOP", ""] -> [w426] mode=indexing
                      n192 = Enqueue Element(queue=w428, element=w426) -> (queue out=w427:refnum<queue>)  [unwired: 2 in, 2 out]
                    }
                  }
                }
                n193 = Select(t=State_Type_Definitions."True Stop" ("Enum"), s=w412, f=State_Type_Definitions."Task 1" ("Enum")) -> (s? t:f=w416:u16)
              }
              frame "Exit" {
                n194 = for {
                  shift-right: [w435] -> w430
                  shift-left: w431 -> [w436]
                  tunnel: string[] ["STOP", "RESET ENCODERS", "RESET YAW", ""] -> [w434] mode=indexing
                  n195 = Enqueue Element(queue=w436, element=w434) -> (queue out=w435:refnum<queue>)  [unwired: 2 in, 2 out]
                }
              }
            }
          }
          frame 8 {
            # ">> Stepper height reeached >>"
            # ">>> yStepper command>>>"
            # ">> Manual override >>"
            n196 = Dequeue Element(queue=w440, timeout in ms (-1)=w439, error in (no error)=w438) -> (element=w449:T7)  [unwired: 3 out]
            n197 = Equal?(x=w442, y=u8 80) -> (x = y?=w447:bool)
            n198 = case shown="\"None\", Default" w449 {
              tunnel: [w460 State_Type_Definitions."True Stop" ("Enum")] -> w444
              tunnel: [w458 w475] -> w437
              tunnel: w446 -> [w457 _]
              tunnel: w445 -> [w451 _]
              tunnel: [State_Type_Definitions."Idle" ("Enum") State_Type_Definitions."Shutdown" ("Enum")] -> w443
              tunnel: w447 -> [w450 _]
              frame "None", Default {
                # ">> WIill proceed to part ii if not manual override >>"
                # ">>If ENABLE or Trigger is set to true>>"
                n199 = Or(x=w450, y=w451) -> (x .or. y?=w452:bool)
                n200 = case shown="True" w450 {
                  tunnel: [w463 w469] -> w458
                  tunnel: w457 -> [w462 w468]
                  frame False {
                    n201 = for {
                      shift-right: [w465] -> w463
                      shift-left: w462 -> [w466]
                      tunnel: string[] ["Z STEPPER CAM HEIGHT", "READ STEPPER VALUES"] ("element") -> [w464] mode=indexing
                      n202 = Enqueue Element(queue=w466, element=w464) -> (queue out=w465:refnum<queue>)  [unwired: 2 in, 2 out]
                    }
                  }
                  frame True {
                    n203 = for {
                      shift-right: [w471] -> w469
                      shift-left: w468 -> [w472]
                      tunnel: string[] ["ARDUINO - ULTRASONIC", "READ ULTRASONIC", "", "", "", ""] -> [w470] mode=indexing
                      n204 = Enqueue Element(queue=w472, element=w470) -> (queue out=w471:refnum<queue>)  [unwired: 2 in, 2 out]
                    }
                  }
                }
                n205 = Select(t=State_Type_Definitions."True Stop" ("Enum"), s=w451, f=State_Type_Definitions."Task 2:Sensor Mode" ("Enum")) -> (s? t:f=w454:T6)
                n206 = Select(t=w454, s=w452, f=State_Type_Definitions."Task 2:Raise Arm" ("Enum")) -> (s? t:f=w460:T6)
              }
              frame "Exit" {
                n207 = for {
                  shift-right: [w478] -> w475
                  shift-left: _ -> [w479]
                  tunnel: string[] ["STOP", "RESET ENCODERS", "RESET YAW", ""] -> [w477] mode=indexing
                  n208 = Enqueue Element(queue=w479, element=w477) -> (queue out=w478:refnum<queue>)  [unwired: 2 in, 2 out]
                }
              }
            }
          }
          frame 9 {
            w494 = u8 20 ("y")
            # ">>> yStepper command>>>"
            # ">>Object detected>>"
            n209 = Dequeue Element(queue=w486, timeout in ms (-1)=w485, error in (no error)=w484) -> (element=w495:T7)  [unwired: 3 out]
            n210 = Less?(x=w482, y=w494) -> (x < y?=w493:bool)
            n211 = Less?(x=w481, y=w494) -> (x < y?=w492:bool)
            n212 = Or(x=w493, y=w492) -> (x .or. y?=w491:bool)
            "Obstacle detected" <- w491
            n213 = case shown="\"None\", Default" w495 {
              tunnel: w491 -> [w498 _]
              tunnel: [w505 State_Type_Definitions."True Stop" ("Enum")] -> w490
              tunnel: w483 -> [w497 _]
              tunnel: w487 -> [w504 w521]
              tunnel: [w503 w522] -> w489
              tunnel: [State_Type_Definitions."Idle" ("Enum") State_Type_Definitions."Shutdown" ("Enum")] -> w488
              frame "None", Default {
                n214 = case shown="True" w498 {
                  tunnel: w504 -> [w508 w515]
                  tunnel: [w509 w514] -> w503
                  frame False {
                    n215 = for {
                      tunnel: string[] ["READ ULTRASONIC", "STOP"] ("element") -> [w510] mode=indexing
                      shift-right: [w512] -> w509
                      shift-left: w508 -> [w511]
                      n216 = Enqueue Element(queue=w511, element=w510) -> (queue out=w512:refnum<queue>)  [unwired: 2 in, 2 out]
                    }
                  }
                  frame True {
                    n217 = for {
                      shift-right: [w517] -> w514
                      shift-left: w515 -> [w518]
                      tunnel: string[] ["SET TIMER 2", "READ NAVX", ""] -> [w516] mode=indexing
                      n218 = Enqueue Element(queue=w518, element=w516) -> (queue out=w517:refnum<queue>)  [unwired: 2 in, 2 out]
                    }
                  }
                }
                n219 = Or(x=w498, y=w497) -> (x .or. y?=w496:bool)
                n220 = Select(t=State_Type_Definitions."True Stop" ("Enum"), s=w497, f=State_Type_Definitions."Task 2:Reverse Mode" ("Enum")) -> (s? t:f=w499:T6)
                n221 = Select(t=w499, s=w496, f=State_Type_Definitions."Task 2:Sensor Mode" ("Enum")) -> (s? t:f=w505:T6)
              }
              frame "Exit" {
                n222 = for {
                  shift-right: [w525] -> w522
                  shift-left: w521 -> [w526]
                  tunnel: string[] ["STOP", "RESET ENCODERS", "RESET YAW", "ARDUINO MODE 0"] -> [w524] mode=indexing
                  n223 = Enqueue Element(queue=w526, element=w524) -> (queue out=w525:refnum<queue>)  [unwired: 2 in, 2 out]
                }
              }
            }
          }
          frame 10 {
            # ">>> yStepper command>>>"
            n224 = Dequeue Element(queue=w533, timeout in ms (-1)=w534, error in (no error)=w535) -> (element=w537:T7)  [unwired: 3 out]
            n225 = case shown="\"None\", Default" w537 {
              tunnel: [w547 State_Type_Definitions."True Stop" ("Enum")] -> w529
              tunnel: w536 -> [w540 _]
              tunnel: w532 -> [w546 w563]
              tunnel: [w545 w564] -> w528
              tunnel: [State_Type_Definitions."Idle" ("Enum") State_Type_Definitions."Shutdown" ("Enum")] -> w530
              tunnel: w527 -> [w538 _]
              frame "None", Default {
                n226 = case shown="True" w538 {
                  tunnel: w546 -> [w550 w557]
                  tunnel: [w551 w556] -> w545
                  frame False {
                    n227 = for {
                      tunnel: string[] ["START TIMER", "REVERSE", "READ NAVX"] ("element") -> [w552] mode=indexing
                      shift-right: [w554] -> w551
                      shift-left: w550 -> [w553]
                      n228 = Enqueue Element(queue=w553, element=w552) -> (queue out=w554:refnum<queue>)  [unwired: 2 in, 2 out]
                    }
                  }
                  frame True {
                    n229 = for {
                      shift-right: [w559] -> w556
                      shift-left: w557 -> [w560]
                      tunnel: string[] ["STOP", "ARDUINO - ULTRASONIC", "READ ULTRASONIC"] -> [w558] mode=indexing
                      n230 = Enqueue Element(queue=w560, element=w558) -> (queue out=w559:refnum<queue>)  [unwired: 2 in, 2 out]
                    }
                  }
                }
                n231 = Or(x=w538, y=w540) -> (x .or. y?=w539:bool)
                n232 = Select(t=State_Type_Definitions."True Stop" ("Enum"), s=w540, f=State_Type_Definitions."Task 2:Sensor Mode" ("Enum")) -> (s? t:f=w541:T6)
                n233 = Select(t=w541, s=w539, f=State_Type_Definitions."Task 2:Reverse Mode" ("Enum")) -> (s? t:f=w547:T6)
              }
              frame "Exit" {
                n234 = for {
                  shift-right: [w567] -> w564
                  shift-left: w563 -> [w568]
                  tunnel: string[] ["STOP", "RESET ENCODERS", "RESET YAW", "ARDUINO MODE 0"] -> [w566] mode=indexing
                  n235 = Enqueue Element(queue=w568, element=w566) -> (queue out=w567:refnum<queue>)  [unwired: 2 in, 2 out]
                }
              }
            }
          }
          frame 11 {
            # ">>> yStepper command>>>"
            n236 = Dequeue Element(queue=w582, timeout in ms (-1)=w581, error in (no error)=w580) -> (element=w571:T7)  [unwired: 3 out]
            n237 = Greater?(x=w579, y=160.0) -> (0:w576:bool)
            n238 = Or(x=w576, y=w577) -> (x .or. y?=w572:bool)
            n239 = case shown="\"None\", Default" w571 {
              tunnel: w572 -> [w585 _]
              tunnel: [w589 State_Type_Definitions."True Stop" ("Enum")] -> w573
              tunnel: w575 -> [w586 w605]
              tunnel: [w584 w604] -> w574
              tunnel: [State_Type_Definitions."Idle" ("Enum") State_Type_Definitions."Shutdown" ("Enum")] -> w570
              frame "None", Default {
                n240 = case shown="False" w585 {
                  tunnel: w586 -> [w592 w598]
                  tunnel: [w591 w596] -> w584
                  frame False {
                    n241 = for {
                      shift-right: [w594] -> w591
                      shift-left: w592 -> [w595]
                      tunnel: string[] ["READ ENCODERS", "R-ACW"] ("element") -> [w593] mode=indexing
                      n242 = Enqueue Element(queue=w595, element=w593) -> (queue out=w594:refnum<queue>)  [unwired: 2 in, 2 out]
                    }
                  }
                  frame True {
                    n243 = for {
                      shift-right: [w600] -> w596
                      shift-left: w598 -> [w601]
                      tunnel: string[] ["RESET YAW", "RESET ENCODERS", "STOP", "ARDUINO MODE 0"] -> [w599] mode=indexing
                      n244 = Enqueue Element(queue=w601, element=w599) -> (queue out=w600:refnum<queue>)  [unwired: 2 in, 2 out]
                    }
                  }
                }
                n245 = Select(t=State_Type_Definitions."True Stop" ("Enum"), s=w585, f=State_Type_Definitions."Task 3" ("Enum")) -> (s? t:f=w589:T6)
              }
              frame "Exit" {
                n246 = for {
                  shift-right: [w608] -> w604
                  shift-left: w605 -> [w609]
                  tunnel: string[] ["STOP", "RESET ENCODERS", "RESET YAW", ""] -> [w607] mode=indexing
                  n247 = Enqueue Element(queue=w609, element=w607) -> (queue out=w608:refnum<queue>)  [unwired: 2 in, 2 out]
                }
              }
            }
          }
          frame 12 {
            # ">> Stepper height reeached >>"
            # ">>> yStepper command>>>"
            # ">> Manual override >>"
            n248 = Dequeue Element(queue=w621, timeout in ms (-1)=w620, error in (no error)=w619) -> (element=w618:T7)  [unwired: 3 out]
            n249 = Equal?(x=w612, y=u8 80) -> (x = y?=w610:bool)
            n250 = case shown="\"Exit\"" w618 {
              tunnel: [w633 State_Type_Definitions."True Stop" ("Enum")] -> w617
              tunnel: [w631 w649] -> w616
              tunnel: w622 -> [w630 w646]
              tunnel: w615 -> [w624 _]
              tunnel: [State_Type_Definitions."Idle" ("Enum") State_Type_Definitions."Shutdown" ("Enum")] -> w614
              tunnel: w610 -> [w623 _]
              frame "None", Default {
                # ">> WIill proceed to part ii if not manual override >>"
                # ">>If ENABLE or Trigger is set to true>>"
                n251 = Or(x=w623, y=w624) -> (x .or. y?=w625:bool)
                n252 = case shown="False" w623 {
                  tunnel: [w636 w642] -> w631
                  tunnel: w630 -> [w635 w641]
                  frame False {
                    n253 = for {
                      shift-right: [w638] -> w636
                      shift-left: w635 -> [w639]
                      tunnel: string[] ["Z STEPPER CAM HEIGHT", "READ STEPPER VALUES"] ("element") -> [w637] mode=indexing
                      n254 = Enqueue Element(queue=w639, element=w637) -> (queue out=w638:refnum<queue>)  [unwired: 2 in, 2 out]
                    }
                  }
                  frame True {
                    n255 = for {
                      shift-right: [w644] -> w642
                      shift-left: w641 -> [w645]
                      tunnel: string[] ["ARDUINO - ULTRASONIC", "READ ULTRASONIC", "FORWARD", "", "", ""] -> [w643] mode=indexing
                      n256 = Enqueue Element(queue=w645, element=w643) -> (queue out=w644:refnum<queue>)  [unwired: 2 in, 2 out]
                    }
                  }
                }
                n257 = Select(t=State_Type_Definitions."True Stop" ("Enum"), s=w624, f=State_Type_Definitions."Task 4_B" ("Enum")) -> (s? t:f=w627:T6)
                n258 = Select(t=w627, s=w625, f=State_Type_Definitions."Task 4_A" ("Enum")) -> (s? t:f=w633:T6)
              }
              frame "Exit" {
                n259 = for {
                  shift-right: [w652] -> w649
                  shift-left: w646 -> [w653]
                  tunnel: string[] ["STOP", "RESET ENCODERS", "RESET YAW", ""] -> [w651] mode=indexing
                  n260 = Enqueue Element(queue=w653, element=w651) -> (queue out=w652:refnum<queue>)  [unwired: 2 in, 2 out]
                }
              }
            }
          }
          frame 13 {
            w657 = u8 20
            # ">> Path blocked >>"
            # ">>> yStepper command>>>"
            # ">> Manual override >>"
            n261 = Dequeue Element(queue=w666, timeout in ms (-1)=w665, error in (no error)=w664) -> (element=w663:T7)  [unwired: 3 out]
            n262 = Less?(x=w659, y=w657) -> (x < y?=w654:bool)
            n263 = Less?(x=w658, y=w657) -> (x < y?=w655:bool)
            n264 = And(x=w655, y=w654) -> (x .and. y?=w656:bool)
            n265 = case shown="\"None\", Default" w663 {
              tunnel: [w680 State_Type_Definitions."True Stop" ("Enum")] -> w668
              tunnel: [w678 w695] -> w669
              tunnel: w662 -> [w677 _]
              tunnel: w667 -> [w671 _]
              tunnel: [State_Type_Definitions."Idle" ("Enum") State_Type_Definitions."Shutdown" ("Enum")] -> w661
              tunnel: w656 -> [w670 _]
              frame "None", Default {
                # ">> Manual override forces program to true stop >>"
                # ">>If ENABLE or Trigger is set to true>>"
                n266 = Or(x=w670, y=w671) -> (x .or. y?=w676:bool)
                n267 = case shown="False" w670 {
                  tunnel: [w683 w688] -> w678
                  tunnel: w677 -> [w682 w687]
                  frame False {
                    n268 = for {
                      shift-right: [w685] -> w683
                      shift-left: w682 -> [w686]
                      tunnel: string[] ["FORWARD", "READ ULTRASONIC", "READ NAVX"] ("element") -> [w684] mode=indexing
                      n269 = Enqueue Element(queue=w686, element=w684) -> (queue out=w685:refnum<queue>)  [unwired: 2 in, 2 out]
                    }
                  }
                  frame True {
                    n270 = for {
                      shift-right: [w691] -> w688
                      shift-left: w687 -> [w692]
                      tunnel: string[] ["STOP", "RESET YAW", "RESET ENCODERS", "RESET FLAGS"] -> [w690] mode=indexing
                      n271 = Enqueue Element(queue=w692, element=w690) -> (queue out=w691:refnum<queue>)  [unwired: 2 in, 2 out]
                    }
                  }
                }
                n272 = Select(t=State_Type_Definitions."True Stop" ("Enum"), s=w671, f=State_Type_Definitions."Task 4_C" ("Enum")) -> (s? t:f=w673:T6)
                n273 = Select(t=w673, s=w676, f=State_Type_Definitions."Task 4_B" ("Enum")) -> (s? t:f=w680:T6)
              }
              frame "Exit" {
                n274 = for {
                  shift-right: [w698] -> w695
                  shift-left: _ -> [w699]
                  tunnel: string[] ["STOP", "RESET ENCODERS", "RESET YAW", ""] -> [w697] mode=indexing
                  n275 = Enqueue Element(queue=w699, element=w697) -> (queue out=w698:refnum<queue>)  [unwired: 2 in, 2 out]
                }
              }
            }
          }
          frame 14 {
            w709 = u8 20
            # ">> xDistance travelled>>"
            # ">> Path NOT blocked >>"
            # ">>> yStepper command>>>"
            # ">> Manual override >>"
            n276 = Dequeue Element(queue=w719, timeout in ms (-1)=w712, error in (no error)=w711) -> (element=w713:T7)  [unwired: 3 out]
            n277 = Greater?(x=w701, y=w709) -> (0:w707:bool)
            n278 = Greater?(x=w706, y=80.0) -> (0:w704:bool)
            n279 = Greater?(x=w700, y=w709) -> (0:w708:bool)
            n280 = And(x=w708, y=w707) -> (x .and. y?=w703:bool)
            n281 = And(x=w704, y=w703) -> (x .and. y?=w702:bool)
            n282 = case shown="\"None\", Default" w713 {
              tunnel: [w730 State_Type_Definitions."True Stop" ("Enum")] -> w716
              tunnel: [w728 w746] -> w715
              tunnel: w718 -> [w727 w743]
              tunnel: w717 -> [w721 _]
              tunnel: [State_Type_Definitions."Idle" ("t") State_Type_Definitions."Shutdown" ("Enum")] -> w714
              tunnel: w702 -> [w720 _]
              frame "None", Default {
                # ">> Manual override forces program to true stop >>"
                # ">>If ENABLE or Trigger is set to true>>"
                n283 = Or(x=w720, y=w721) -> (x .or. y?=w726:bool)
                n284 = case shown="False" w720 {
                  tunnel: [w733 w738] -> w728
                  tunnel: w727 -> [w731 w737]
                  frame False {
                    n285 = for {
                      shift-right: [w735] -> w733
                      shift-left: w731 -> [w736]
                      tunnel: string[] ["RIGHT", "READ NAVX", "READ ENCODERS", "READ ULTRASONIC"] ("element") -> [w734] mode=indexing
                      n286 = Enqueue Element(queue=w736, element=w734) -> (queue out=w735:refnum<queue>)  [unwired: 2 in, 2 out]
                    }
                  }
                  frame True {
                    n287 = for {
                      shift-right: [w741] -> w738
                      shift-left: w737 -> [w742]
                      tunnel: string[] ["STOP", "RESET YAW", "RESET ENCODERS", "ARDUINO - ULTRASONIC"] -> [w740] mode=indexing
                      n288 = Enqueue Element(queue=w742, element=w740) -> (queue out=w741:refnum<queue>)  [unwired: 2 in, 2 out]
                    }
                  }
                }
                n289 = Select(t=State_Type_Definitions."True Stop" ("Enum"), s=w721, f=State_Type_Definitions."Task 4_D" ("Enum")) -> (s? t:f=w722:T6)
                n290 = Select(t=w722, s=w726, f=State_Type_Definitions."Task 4_C" ("Enum")) -> (s? t:f=w730:T6)
              }
              frame "Exit" {
                n291 = for {
                  shift-right: [w749] -> w746
                  shift-left: w743 -> [w750]
                  tunnel: string[] ["STOP", "RESET ENCODERS", "RESET YAW", ""] -> [w748] mode=indexing
                  n292 = Enqueue Element(queue=w750, element=w748) -> (queue out=w749:refnum<queue>)  [unwired: 2 in, 2 out]
                }
              }
            }
          }
          frame 15 {
            w769 = u8 20
            # ">> yDistance travelled>>"
            # ">> Path blocked >>"
            # ">>> yStepper command>>>"
            # ">> Manual override >>"
            n293 = Dequeue Element(queue=w760, timeout in ms (-1)=w759, error in (no error)=w758) -> (element=w770:T7)  [unwired: 3 out]
            n294 = Less?(x=w753, y=w769) -> (x < y?=w767:bool)
            n295 = Greater?(x=w757, y=200.0) -> (0:w765:bool)
            n296 = Less?(x=w752, y=w769) -> (x < y?=w768:bool)
            n297 = And(x=w768, y=w767) -> (x .and. y?=w764:bool)
            n298 = Or(x=w765, y=w764) -> (x .or. y?=w763:bool)
            n299 = case shown="\"None\", Default" w770 {
              tunnel: [w781 State_Type_Definitions."True Stop" ("Enum")] -> w756
              tunnel: [w779 w797] -> w754
              tunnel: w761 -> [w778 w794]
              tunnel: w762 -> [w772 _]
              tunnel: [State_Type_Definitions."Idle" ("t") State_Type_Definitions."Shutdown" ("Enum")] -> w755
              tunnel: w763 -> [w771 _]
              frame "None", Default {
                # ">> Manual override forces program to true stop >>"
                # ">>If ENABLE or Trigger is set to true>>"
                n300 = Or(x=w771, y=w772) -> (x .or. y?=w777:bool)
                n301 = case shown="True" w771 {
                  tunnel: [w784 w789] -> w779
                  tunnel: w778 -> [w782 w788]
                  frame False {
                    n302 = for {
                      shift-right: [w786] -> w784
                      shift-left: w782 -> [w787]
                      tunnel: string[] ["FORWARD", "READ NAVX", "READ ENCODERS", "READ ULTRASONIC"] ("element") -> [w785] mode=indexing
                      n303 = Enqueue Element(queue=w787, element=w785) -> (queue out=w786:refnum<queue>)  [unwired: 2 in, 2 out]
                    }
                  }
                  frame True {
                    n304 = for {
                      shift-right: [w792] -> w789
                      shift-left: w788 -> [w793]
                      tunnel: string[] ["STOP", "RESET YAW", "RESET ENCODERS", "RESET FLAGS"] -> [w791] mode=indexing
                      n305 = Enqueue Element(queue=w793, element=w791) -> (queue out=w792:refnum<queue>)  [unwired: 2 in, 2 out]
                    }
                  }
                }
                n306 = Select(t=State_Type_Definitions."True Stop" ("Enum"), s=w772, f=State_Type_Definitions."True Stop" ("Enum")) -> (s? t:f=w773:T6)
                n307 = Select(t=w773, s=w777, f=State_Type_Definitions."Task 4_D" ("Enum")) -> (s? t:f=w781:T6)
              }
              frame "Exit" {
                n308 = for {
                  shift-right: [w800] -> w797
                  shift-left: w794 -> [w801]
                  tunnel: string[] ["STOP", "RESET ENCODERS", "RESET YAW", ""] -> [w799] mode=indexing
                  n309 = Enqueue Element(queue=w801, element=w799) -> (queue out=w800:refnum<queue>)  [unwired: 2 in, 2 out]
                }
              }
            }
          }
          frame 15 {
            # ">>> yStepper command>>>"
            # ">> Manual override >>"
            n310 = Dequeue Element(queue=w810, timeout in ms (-1)=w809, error in (no error)=w811) -> (element=w808:T7)  [unwired: 3 out]
            n311 = Equal?(x=w807, y=u8 80) -> (x = y?=w805:bool)
            n312 = case shown="\"None\", Default" w808 {
              tunnel: [w821 State_Type_Definitions."True Stop" ("Enum")] -> w812
              tunnel: [w824 w841] -> w813
              tunnel: [State_Type_Definitions."Idle" ("Enum") State_Type_Definitions."Shutdown" ("Enum")] -> w814
              tunnel: w805 -> [w820 _]
              tunnel: w804 -> [w819 _]
              tunnel: w803 -> [w815 w838]
              frame "None", Default {
                # "Stays in Task 5_A until stepper reaches desired \nheight"
                # "T: Go back to idle, F: Continue with task\""
                # ">> Manual override >>"
                n313 = case shown="True" w820 {
                  tunnel: [w828 w834] -> w824
                  tunnel: w815 -> [w826 w832]
                  frame False {
                    n314 = for {
                      tunnel: string[] ["Z STEPPER CAM HEIGHT", "READ STEPPER VALUES"] ("element") -> [w829] mode=indexing
                      shift-right: [w831] -> w828
                      shift-left: w826 -> [w830]
                      n315 = Enqueue Element(queue=w830, element=w829) -> (queue out=w831:refnum<queue>)  [unwired: 2 in, 2 out]
                    }
                  }
                  frame True {
                    n316 = for {
                      shift-right: [w836] -> w834
                      shift-left: w832 -> [w837]
                      tunnel: string[] ["ARDUINO - ULTRASONIC", "READ ULTRASONIC", ""] -> [w835] mode=indexing
                      n317 = Enqueue Element(queue=w837, element=w835) -> (queue out=w836:refnum<queue>)  [unwired: 2 in, 2 out]
                    }
                  }
                }
                n318 = Or(x=w820, y=w819) -> (x .or. y?=w822:bool)
                n319 = Select(t=State_Type_Definitions."True Stop" ("Enum"), s=w819, f=State_Type_Definitions."Task 5 _B" ("Enum")) -> (s? t:f=w816:u16)
                n320 = Select(t=w816, s=w822, f=State_Type_Definitions."Task 5_A" ("Enum")) -> (s? t:f=w821:u16)
              }
              frame "Exit" {
                n321 = for {
                  shift-right: [w844] -> w841
                  shift-left: w838 -> [w845]
                  tunnel: string[] ["STOP", "RESET ENCODERS", "RESET YAW", "ARDUINO MODE 0"] -> [w843] mode=indexing
                  n322 = Enqueue Element(queue=w845, element=w843) -> (queue out=w844:refnum<queue>)  [unwired: 2 in, 2 out]
                }
              }
            }
          }
          frame 16 {
            w851 = u8 20 ("y")
            # ">>> yStepper command>>>"
            n323 = Less?(x=w848, y=w851) -> (x < y?=w849:bool)
            n324 = Dequeue Element(queue=w855, timeout in ms (-1)=w854, error in (no error)=w856) -> (element=w853:T7)  [unwired: 3 out]
            n325 = Less?(x=w847, y=w851) -> (x < y?=w850:bool)
            n326 = And(x=w850, y=w849) -> (x .and. y?=w846:bool)
            n327 = case shown="\"Exit\"" w853 {
              tunnel: [w868 State_Type_Definitions."True Stop" ("Enum")] -> w858
              tunnel: [w871 w888] -> w857
              tunnel: [State_Type_Definitions."Idle" ("Enum") State_Type_Definitions."Shutdown" ("Enum")] -> w859
              tunnel: w861 -> [w867 _]
              tunnel: w860 -> [w863 w885]
              tunnel: w846 -> [w862 _]
              frame "None", Default {
                # "Stays in Task 5_B to capture image over 5 seconds"
                # "T: Go back to idle, F: Continue with task\""
                # ">> Manual override >>"
                n328 = case shown="False" w862 {
                  tunnel: [w875 w881] -> w871
                  tunnel: w863 -> [w873 w879]
                  frame False {
                    n329 = for {
                      tunnel: string[] ["FORWARD", "READ ULTRASONIC", "READ NAVX"] ("element") -> [w876] mode=indexing
                      shift-right: [w878] -> w875
                      shift-left: w873 -> [w877]
                      n330 = Enqueue Element(queue=w877, element=w876) -> (queue out=w878:refnum<queue>)  [unwired: 2 in, 2 out]
                    }
                  }
                  frame True {
                    n331 = for {
                      shift-right: [w883] -> w881
                      shift-left: w879 -> [w884]
                      tunnel: string[] ["STOP", "RESET ENCODERS", "OPEN LOG CAM", "SET TIMER"] -> [w882] mode=indexing
                      n332 = Enqueue Element(queue=w884, element=w882) -> (queue out=w883:refnum<queue>)  [unwired: 2 in, 2 out]
                    }
                  }
                }
                n333 = Or(x=w862, y=w867) -> (x .or. y?=w869:bool)
                n334 = Select(t=State_Type_Definitions."True Stop" ("Enum"), s=w867, f=State_Type_Definitions."Task 5_C" ("Enum")) -> (s? t:f=w864:u16)
                n335 = Select(t=w864, s=w869, f=State_Type_Definitions."Task 5 _B" ("Enum")) -> (s? t:f=w868:u16)
              }
              frame "Exit" {
                n336 = for {
                  shift-right: [w891] -> w888
                  shift-left: w885 -> [w892]
                  tunnel: string[] ["STOP", "RESET ENCODERS", "RESET YAW", "ARDUINO MODE 0"] -> [w890] mode=indexing
                  n337 = Enqueue Element(queue=w892, element=w890) -> (queue out=w891:refnum<queue>)  [unwired: 2 in, 2 out]
                }
              }
            }
          }
          frame 17 {
            # ">>> yStepper command>>>"
            # ">> Manual override >>"
            n338 = Dequeue Element(queue=w901, timeout in ms (-1)=w900, error in (no error)=w899) -> (element=w898:T7)  [unwired: 3 out]
            n339 = case shown="\"None\", Default" w898 {
              tunnel: [w908 State_Type_Definitions."True Stop" ("Enum")] -> w903
              tunnel: [w911 w928] -> w896
              tunnel: [State_Type_Definitions."Idle" ("Enum") State_Type_Definitions."Shutdown" ("Enum")] -> w895
              tunnel: w897 -> [w905 _]
              tunnel: w902 -> [w907 w925]
              tunnel: w893 -> [w904 _]
              frame "None", Default {
                # ">> Is time up? >>"
                # "Determines if object is in range to pick up"
                # ">> Manual override >>"
                n340 = case shown="False" w904 {
                  tunnel: [w915 w921] -> w911
                  tunnel: w907 -> [w913 w919]
                  frame False {
                    n341 = for {
                      tunnel: string[] ["CAM ACQ", "START TIMER"] ("element") -> [w916] mode=indexing
                      shift-right: [w918] -> w915
                      shift-left: w913 -> [w917]
                      n342 = Enqueue Element(queue=w917, element=w916) -> (queue out=w918:refnum<queue>)  [unwired: 2 in, 2 out]
                    }
                  }
                  frame True {
                    n343 = for {
                      shift-right: [w923] -> w921
                      shift-left: w919 -> [w924]
                      tunnel: string[] ["CAM CLOSE", "PROCESS IMAGE"] -> [w922] mode=indexing
                      n344 = Enqueue Element(queue=w924, element=w922) -> (queue out=w923:refnum<queue>)  [unwired: 2 in, 2 out]
                    }
                  }
                }
                n345 = Or(x=w904, y=w905) -> (x .or. y?=w909:bool)
                n346 = Select(t=State_Type_Definitions."Task 5_D" ("Enum"), s=w909, f=State_Type_Definitions."Task 5_D" ("Enum")) -> (s? t:f=w908:T24)
              }
              frame "Exit" {
                n347 = for {
                  shift-right: [w931] -> w928
                  shift-left: w925 -> [w932]
                  tunnel: string[] ["STOP", "RESET ENCODERS", "RESET YAW", "ARDUINO MODE 0"] -> [w930] mode=indexing
                  n348 = Enqueue Element(queue=w932, element=w930) -> (queue out=w931:refnum<queue>)  [unwired: 2 in, 2 out]
                }
              }
            }
          }
          frame 18 {
            # ">>> yStepper command>>>"
            n349 = Dequeue Element(queue=w938, timeout in ms (-1)=w937, error in (no error)=w936) -> (element=w935:T7)  [unwired: 3 out]
            n350 = case shown="\"None\", Default" w935 {
              tunnel: [w950 State_Type_Definitions."True Stop" ("Enum")] -> w942
              tunnel: [w953 w970] -> w941
              tunnel: [State_Type_Definitions."Idle" ("Enum") State_Type_Definitions."Shutdown" ("Enum")] -> w943
              tunnel: w939 -> [w949 _]
              tunnel: w940 -> [w945 w967]
              tunnel: w933 -> [w944 _]
              frame "None", Default {
                # ">> T: Breaks out of state loop; F: Stays in loop>>"
                # ">> Manual override >>"
                # ">> Checks if object is detected>>"
                # "Stays in Task 5D until the object is detected"
                # "T: Go back to idle, F: Continue with task\""
                # ">> Manual override >>"
                n351 = case shown="False" w944 {
                  tunnel: [w957 w963] -> w953
                  tunnel: w945 -> [w955 w961]
                  frame False {
                    n352 = for {
                      tunnel: string[] ["PROCESS IMAGE", "", ""] ("element") -> [w958] mode=indexing
                      shift-right: [w960] -> w957
                      shift-left: w955 -> [w959]
                      n353 = Enqueue Element(queue=w959, element=w958) -> (queue out=w960:refnum<queue>)  [unwired: 2 in, 2 out]
                    }
                  }
                  frame True {
                    n354 = for {
                      shift-right: [w965] -> w963
                      shift-left: w961 -> [w966]
                      tunnel: string[] ["DISPOSE BUFFERS", "CAM CLOSE", ""] -> [w964] mode=indexing
                      n355 = Enqueue Element(queue=w966, element=w964) -> (queue out=w965:refnum<queue>)  [unwired: 2 in, 2 out]
                    }
                  }
                }
                n356 = Or(x=w944, y=w949) -> (x .or. y?=w951:bool)
                n357 = Select(t=State_Type_Definitions."True Stop" ("Enum"), s=w949, f=State_Type_Definitions."True Stop" ("Enum")) -> (s? t:f=w946:T6)
                n358 = Select(t=w946, s=w951, f=State_Type_Definitions."Task 5_D" ("Enum")) -> (s? t:f=w950:u16)
              }
              frame "Exit" {
                n359 = for {
                  shift-right: [w973] -> w970
                  shift-left: w967 -> [w974]
                  tunnel: string[] ["STOP", "RESET ENCODERS", "RESET YAW", "ARDUINO MODE 0"] -> [w972] mode=indexing
                  n360 = Enqueue Element(queue=w974, element=w972) -> (queue out=w973:refnum<queue>)  [unwired: 2 in, 2 out]
                }
              }
            }
          }
          frame 24 {
            # ">>> yStepper command>>>"
            n361 = Dequeue Element(queue=w982, timeout in ms (-1)=w981, error in (no error)=w980) -> (element=w987:T7)  [unwired: 3 out]
            n362 = Equal?(x=w978, y=u8 80) -> (x = y?=w977:bool)
            n363 = case shown="\"None\", Default" w987 {
              tunnel: [w994 State_Type_Definitions."True Stop" ("Enum")] -> w985
              tunnel: [w993 w1011] -> w984
              tunnel: [State_Type_Definitions."Idle" ("Enum") State_Type_Definitions."Shutdown" ("Enum")] -> w986
              tunnel: w983 -> [w989 _]
              tunnel: w979 -> [w991 _]
              tunnel: w977 -> [w988 _]
              frame "None", Default {
                n364 = case shown="False" w988 {
                  tunnel: [w999 w1005] -> w993
                  tunnel: w991 -> [w997 w1003]
                  frame False {
                    n365 = for {
                      tunnel: string[] ["Z STEPPER CAM HEIGHT", "READ STEPPER VALUES"] ("element") -> [w1000] mode=indexing
                      shift-right: [w1002] -> w999
                      shift-left: w997 -> [w1001]
                      n366 = Enqueue Element(queue=w1001, element=w1000) -> (queue out=w1002:refnum<queue>)  [unwired: 2 in, 2 out]
                    }
                  }
                  frame True {
                    n367 = for {
                      shift-right: [w1007] -> w1005
                      shift-left: w1003 -> [w1008]
                      tunnel: string[] ["CAM ACQ", "OPEN LOG CAM"] -> [w1006] mode=indexing
                      n368 = Enqueue Element(queue=w1008, element=w1006) -> (queue out=w1007:refnum<queue>)  [unwired: 2 in, 2 out]
                    }
                  }
                }
                n369 = Or(x=w988, y=w989) -> (x .or. y?=w990:bool)
                n370 = Select(t=State_Type_Definitions."Task 6_B" ("Enum"), s=w990, f=State_Type_Definitions."Task 6_A" ("Enum")) -> (s? t:f=w994:T6)
              }
              frame "Exit" {
                n371 = for {
                  shift-right: [w1014] -> w1011
                  shift-left: _ -> [w1015]
                  tunnel: string[] ["STOP", "RESET ENCODERS", "RESET YAW", "ARDUINO MODE 0"] -> [w1013] mode=indexing
                  n372 = Enqueue Element(queue=w1015, element=w1013) -> (queue out=w1014:refnum<queue>)  [unwired: 2 in, 2 out]
                }
              }
            }
          }
          frame 25 {
            # ">>> yStepper command>>>"
            n373 = Dequeue Element(queue=w1025, timeout in ms (-1)=w1023, error in (no error)=w1024) -> (element=w1022:T7)  [unwired: 3 out]
            n374 = case shown="\"None\", Default" w1022 {
              tunnel: [w1032 State_Type_Definitions."True Stop" ("Enum")] -> w1018
              tunnel: [w1031 w1050] -> w1026
              tunnel: [State_Type_Definitions."Idle" ("Enum") State_Type_Definitions."Shutdown" ("Enum")] -> w1019
              tunnel: w1021 -> [w1027 _]
              tunnel: w1020 -> [w1029 _]
              tunnel: w1017 -> [w1028 w1047]
              frame "None", Default {
                # ">> Manual override >>"
                n375 = case shown="True" w1029 {
                  tunnel: [w1037 w1043] -> w1031
                  tunnel: w1028 -> [w1036 w1041]
                  frame False {
                    n376 = for {
                      shift-right: [w1040] -> w1037
                      shift-left: w1036 -> [w1039]
                      tunnel: string[] ["CAM ACQ", "PROCESS IMAGE", "OPEN CLAW"] -> [w1038] mode=indexing
                      n377 = Enqueue Element(queue=w1039, element=w1038) -> (queue out=w1040:refnum<queue>)  [unwired: 2 in, 2 out]
                    }
                  }
                  frame True {
                    n378 = for {
                      shift-right: [w1045] -> w1043
                      shift-left: w1041 -> [w1046]
                      tunnel: string[] ["CAM ACQ", "PROCESS IMAGE", "CLOSE CLAW"] -> [w1044] mode=indexing
                      n379 = Enqueue Element(queue=w1046, element=w1044) -> (queue out=w1045:refnum<queue>)  [unwired: 2 in, 2 out]
                    }
                  }
                }
                n380 = Select(t=State_Type_Definitions."True Stop" ("Enum"), s=w1027, f=State_Type_Definitions."Task 6_B" ("Enum")) -> (s? t:f=w1032:T6)
              }
              frame "Exit" {
                # ">> State after true stop >>"
                # ">> Goes to true stop >>"
                n381 = for {
                  shift-right: [w1053] -> w1050
                  shift-left: w1047 -> [w1054]
                  tunnel: string[] ["STOP", "RESET ENCODERS", "RESET YAW", ""] -> [w1052] mode=indexing
                  n382 = Enqueue Element(queue=w1054, element=w1052) -> (queue out=w1053:refnum<queue>)  [unwired: 2 in, 2 out]
                }
              }
            }
          }
          frame 38 {
            # ">> Stepper height reeached >>"
            # ">>> yStepper command>>>"
            # ">> Manual override >>"
            n383 = Dequeue Element(queue=w1064, timeout in ms (-1)=w1059, error in (no error)=w1063) -> (element=w1067:T7)  [unwired: 3 out]
            n384 = Equal?(x=w1061, y=u8 80) -> (x = y?=w1065:bool)
            n385 = case shown="\"None\", Default" w1067 {
              tunnel: [w1078 State_Type_Definitions."True Stop" ("Enum")] -> w1057
              tunnel: [w1076 w1093] -> w1056
              tunnel: w1060 -> [w1075 _]
              tunnel: w1062 -> [w1069 _]
              tunnel: [State_Type_Definitions."Idle" ("Enum") State_Type_Definitions."Shutdown" ("Enum")] -> w1058
              tunnel: w1065 -> [w1068 _]
              frame "None", Default {
                # ">> WIill proceed to part ii if not manual override >>"
                # ">>If ENABLE or Trigger is set to true>>"
                n386 = Or(x=w1068, y=w1069) -> (x .or. y?=w1070:bool)
                n387 = case shown="True" w1068 {
                  tunnel: [w1081 w1087] -> w1076
                  tunnel: w1075 -> [w1080 w1086]
                  frame False {
                    n388 = for {
                      shift-right: [w1083] -> w1081
                      shift-left: w1080 -> [w1084]
                      tunnel: string[] ["Z STEPPER CAM HEIGHT", "READ STEPPER VALUES"] ("element") -> [w1082] mode=indexing
                      n389 = Enqueue Element(queue=w1084, element=w1082) -> (queue out=w1083:refnum<queue>)  [unwired: 2 in, 2 out]
                    }
                  }
                  frame True {
                    n390 = for {
                      shift-right: [w1089] -> w1087
                      shift-left: w1086 -> [w1090]
                      tunnel: string[] ["ARDUINO - ULTRASONIC", "READ ULTRASONIC", "", "", "", ""] -> [w1088] mode=indexing
                      n391 = Enqueue Element(queue=w1090, element=w1088) -> (queue out=w1089:refnum<queue>)  [unwired: 2 in, 2 out]
                    }
                  }
                }
                n392 = Select(t=State_Type_Definitions."True Stop" ("Enum"), s=w1069, f=State_Type_Definitions."Task 9B: Rotate to Angle" ("Enum")) -> (s? t:f=w1072:T6)
                n393 = Select(t=w1072, s=w1070, f=State_Type_Definitions."Task 9A: Raise Arm" ("Enum")) -> (s? t:f=w1078:T6)
              }
              frame "Exit" {
                n394 = for {
                  shift-right: [w1096] -> w1093
                  shift-left: _ -> [w1097]
                  tunnel: string[] ["STOP", "RESET ENCODERS", "RESET YAW", ""] -> [w1095] mode=indexing
                  n395 = Enqueue Element(queue=w1097, element=w1095) -> (queue out=w1096:refnum<queue>)  [unwired: 2 in, 2 out]
                }
              }
            }
          }
          frame 39 {
            # ">>> yStepper command>>>"
            n396 = Dequeue Element(queue=w1109, timeout in ms (-1)=w1108, error in (no error)=w1107) -> (element=w1111:T7)  [unwired: 3 out]
            n397 = In Range and Coerce(upper limit=305.0, x=w1101, lower limit=295.0) -> (In Range?=w1098:bool)  [unwired: 1 out]
            n398 = case shown="\"None\", Default" w1111 {
              tunnel: w1102 -> [w1114 _]
              tunnel: [w1122 State_Type_Definitions."True Stop" ("Enum")] -> w1104
              tunnel: w1110 -> [w1120 w1138]
              tunnel: [w1119 w1137] -> w1103
              tunnel: [State_Type_Definitions."Idle" ("Enum") State_Type_Definitions."Shutdown" ("Enum")] -> w1105
              tunnel: w1098 -> [w1112 _]
              frame "None", Default {
                n399 = Or(x=w1112, y=w1114) -> (x .or. y?=w1113:bool)
                n400 = case shown="True" w1112 {
                  tunnel: w1120 -> [w1125 w1131]
                  tunnel: [w1124 w1129] -> w1119
                  frame False {
                    n401 = for {
                      shift-right: [w1127] -> w1124
                      shift-left: w1125 -> [w1128]
                      tunnel: string[] ["READ NAVX", "R-ACW"] ("element") -> [w1126] mode=indexing
                      n402 = Enqueue Element(queue=w1128, element=w1126) -> (queue out=w1127:refnum<queue>)  [unwired: 2 in, 2 out]
                    }
                  }
                  frame True {
                    n403 = for {
                      shift-right: [w1133] -> w1129
                      shift-left: w1131 -> [w1134]
                      tunnel: string[] ["STOP", "RESET ENCODERS", "RESET YAW", ""] -> [w1132] mode=indexing
                      n404 = Enqueue Element(queue=w1134, element=w1132) -> (queue out=w1133:refnum<queue>)  [unwired: 2 in, 2 out]
                    }
                  }
                }
                n405 = Select(t=State_Type_Definitions."True Stop" ("Enum"), s=w1114, f=State_Type_Definitions."Task 9C: Rotation alignmnet") -> (s? t:f=w1116:u16)
                n406 = Select(t=w1116, s=w1113, f=State_Type_Definitions."Task 9B: Rotate to Angle" ("Enum")) -> (s? t:f=w1122:u16)
              }
              frame "Exit" {
                n407 = for {
                  shift-right: [w1141] -> w1137
                  shift-left: w1138 -> [w1142]
                  tunnel: string[] ["STOP", "RESET ENCODERS", "RESET YAW", ""] -> [w1140] mode=indexing
                  n408 = Enqueue Element(queue=w1142, element=w1140) -> (queue out=w1141:refnum<queue>)  [unwired: 2 in, 2 out]
                }
              }
            }
          }
          frame 34 {
            # ">>> yStepper command>>>"
            n409 = Dequeue Element(queue=w1151, timeout in ms (-1)=w1150, error in (no error)=w1149) -> (element=w1152:T7)  [unwired: 3 out]
            n410 = case shown="\"None\", Default" w1152 {
              tunnel: w1147 -> [w1153 _]
              tunnel: [w1161 State_Type_Definitions."True Stop" ("Enum")] -> w1144
              tunnel: w1148 -> [w1159 w1177]
              tunnel: [w1158 w1176] -> w1143
              tunnel: [State_Type_Definitions."Idle" ("Enum") State_Type_Definitions."Shutdown" ("Enum")] -> w1146
              frame "None", Default {
                n411 = case shown="True" w1153 {
                  tunnel: w1159 -> [w1164 w1170]
                  tunnel: [w1163 w1168] -> w1158
                  frame False {
                    n412 = for {
                      shift-right: [w1166] -> w1163
                      shift-left: w1164 -> [w1167]
                      tunnel: string[] ["READ IR", "FORWARD - IR ASSIST"] ("element") -> [w1165] mode=indexing
                      n413 = Enqueue Element(queue=w1167, element=w1165) -> (queue out=w1166:refnum<queue>)  [unwired: 2 in, 2 out]
                    }
                  }
                  frame True {
                    n414 = for {
                      shift-right: [w1172] -> w1168
                      shift-left: w1170 -> [w1173]
                      tunnel: string[] ["STOP", "RESET ENCODERS", "RESET YAW", ""] -> [w1171] mode=indexing
                      n415 = Enqueue Element(queue=w1173, element=w1171) -> (queue out=w1172:refnum<queue>)  [unwired: 2 in, 2 out]
                    }
                  }
                }
                n416 = Select(t=State_Type_Definitions."True Stop" ("Enum"), s=w1153, f=State_Type_Definitions."True Stop") -> (s? t:f=w1155:T6)
                n417 = Select(t=w1155, s=w1153, f=State_Type_Definitions."Task 9C: Rotation alignmnet" ("Enum")) -> (s? t:f=w1161:u16)
              }
              frame "Exit" {
                n418 = for {
                  shift-right: [w1180] -> w1176
                  shift-left: w1177 -> [w1181]
                  tunnel: string[] ["STOP", "RESET ENCODERS", "RESET YAW", ""] -> [w1179] mode=indexing
                  n419 = Enqueue Element(queue=w1181, element=w1179) -> (queue out=w1180:refnum<queue>)  [unwired: 2 in, 2 out]
                }
              }
            }
          }
        }
      }
    }
    n420 = local write "Green LED"(w199) -> ()
  }
  n421 = call <vilib>:"DIO Close.vi"("error in (no error)"=w25, "DIO Info In"=w28) -> ()  [unwired: 9 in, 1 out]
  n422 = call <vilib>:"DIO Close.vi"("error in (no error)"=w35, "DIO Info In"=w37) -> ()  [unwired: 9 in, 1 out]
  n423 = call <vilib>:"NavX Close.vi"("error in (no error)"=w6, "NavX Info In"=w5) -> ()  [unwired: 9 in, 1 out]
  n424 = call <vilib>:"DIO Close.vi"("error in (no error)"=w30, "DIO Info In"=w32) -> ()  [unwired: 9 in, 1 out]
  n425 = call <vilib>:"DIO Close.vi"("error in (no error)"=w13, "DIO Info In"=w14) -> ()  [unwired: 9 in, 1 out]
  n426 = call <vilib>:"DIO Close.vi"("error in (no error)"=w8, "DIO Info In"=w9) -> ()  [unwired: 9 in, 1 out]
  n427 = while {
    stop <- w1729 stop-if-true
    n428 = call <vilib>:"RT Get CPU Loads.vi"() -> ("CPU loads"=→"CPU loads":T5[])  [unwired: 10 in, 1 out]
    n429 = Wait (ms)(milliseconds to wait=u32 100) -> ()  [unwired: 1 out]
    n430 = call "FGV Bool.vi"("Init/Read/Write State"=States_for_Action_Engine."Read") -> ("Output node"=w1729:bool)  [unwired: 2 in, 1 out]
  }
  n431 = while {
    stop <- w1733 stop-if-true
    n432 = call "MOTOR CONTROL WITH PID AE.vi"("AE Mode"=MOTOR_CONTROL_WITH_PID_AE_DATA_MODE_TYPE_DEF."Read from AE") -> ("Speed & distance"=→"Speed & distance":T1)  [unwired: 3 in]
    n433 = call "FGV Bool.vi"("Init/Read/Write State"=States_for_Action_Engine."Read") -> ("Output node"=w1733:bool)  [unwired: 2 in, 1 out]
    n434 = Wait (ms)(milliseconds to wait=u32 5) -> ()  [unwired: 1 out]
  }
  n435 = Merge Errors "Merge Errors"(w65, w64) -> (w47:errorcluster)
  n436 = Merge Errors(w51, w47) -> (w46:errorcluster)
  n437 = Destroy User Event(user event=w68, error in=w46) -> ()  [unwired: 1 out]
  n438 = Destroy User Event(user event=w69, error in=w46) -> ()  [unwired: 1 out]
  n439 = Unregister For Events(event registration refnum=w60, error in=w46) -> ()  [unwired: 1 out]
  n440 = Release Queue(queue=w42, error in (no error)=w46) -> (error out=w24:errorcluster)  [unwired: 1 in, 2 out]
  n441 = Release Queue(queue=w59, error in (no error)=w46) -> ()  [unwired: 1 in, 3 out]
  n442 = call <vilib>:"Simple Error Handler.vi"("error in (no error)"=w24) -> ("error out"=w23:errorcluster)  [unwired: 4 in, 4 out]
  n443 = call <vilib>:"Reset myRIO.vi"("error in (no error)"=w23) -> ("error out"=→"error out":errorcluster)  [unwired: 10 in]
